vi "MOCVD_Growth_Sequence_Editor.vi"() -> ()   [LabVIEW 2011]
doc: "This is the top-level Growth Sequence Editor Application, and the only VI that needs to be executed by the end-user to edit and run a growth sequence. This application provides all functions necessary for opening, saving, and editing growth sequence files."
uses:
  low_level_proc/globals.vi
panel:
  out "opening_sequence":bool
  out "Error Out":errorcluster
  out "Total Time":string caption="Total Growth Time:"
  out "Notes":string
  out "Growth Name":string
  out "Operator Name":string
  out "Db Info Set":bool
  in  "Set DB Info":bool
  out "Use Database":bool=TRUE
  out "Log Files Directory":path=path "C:/MOCVD/Log Files"
  in  "Preferences":bool
  in  "Iterations":u32=1 min=1
  out "Delete Event":bool
  out "Current File Path":path
  in  "Save":bool
  out "Application Name":string
  in  "Comment":string
  out "Error Out":errorcluster caption="error out"
  in  "Operating Mode":enum32{"Production", "Debug"}(radio)=enum."Debug"
  in  "View Log":bool
  in  "Resume":bool
  in  "Exit":bool
  in  "New Sequence":bool
  in  "Save As":bool
  in  "Command Tabs":T1(tab)
  in  "Active":bool
  in  "Run":bool
  in  "Flow 1":dbl caption="Flow 1 (sccm)" min=0.0
  in  "Flow 2":dbl caption="Flow 2 (sccm)" min=0.0
  in  "Flow 3":dbl caption="Flow 3 (sccm)" min=0.0
  in  "Flow 4":dbl caption="Flow 4 (sccm)" min=0.0
  in  "Gas_Source_In":bool caption="Gas Source In"
  in  "H2 Flush":bool
  in  "Bubbler In":bool
  in  "H2_Dilute":bool caption="H2 Dilute"
  in  "Remote Flow":bool caption="Remote"
  in  "Spinner":bool
  in  "Heater":bool
  in  "Remote Heater":bool caption="Remote"
  in  "Atm_Exhaust":bool
  in  "Vac_Exhaust":bool
  in  "Remote Vacuum":bool caption="Remote"
  in  "Prompt":string
  in  "API Front Panel":bool
  in  "Move Down":bool
  in  "Move Up":bool
  in  "Copy Event":bool
  in  "Time (s)":dbl min=0.0
  out "Command":string
  in  "Command Sequence":i32[](listbox)
  in  "Delete Event":bool
  in  "Insert Event":bool
  in  "Run Sequence":bool
  in  "Open Sequence":bool
  # "Wait for user input before continuing sequence"
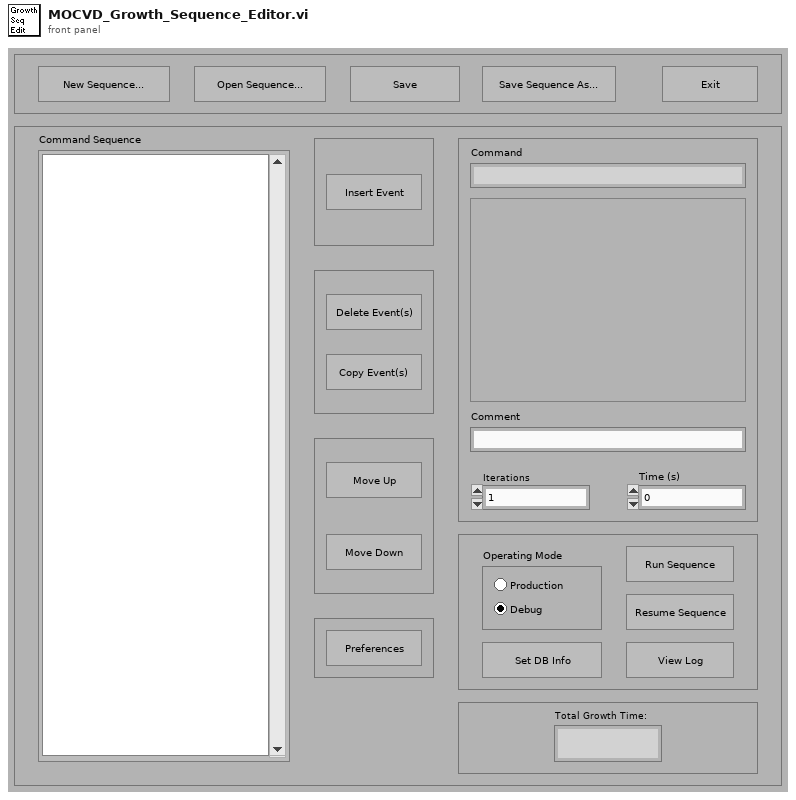
[diagram p1: front panel]
types:
  T1 = enum32{"Default", "Flow", "Heater", "Vacuum", "Wait", "API"}
  T2 = cluster{"Command":string, "Argument List":string[], dbl[], "element":dbl}
  T3 = cluster{"Command":string, "Argument List Out":string[], dbl[], "element":dbl}
  T4 = cluster{"Command":string, string[], dbl[], "element":dbl}
  T5 = enum16{"Discrete", "Continuous", "Instantaneous", "Finite"}
  T6 = cluster{string, "Argument List Out":string[], dbl[], dbl}
  T7 = enum8{"Enabled", "Disabled", "Disabled and Grayed Out"}
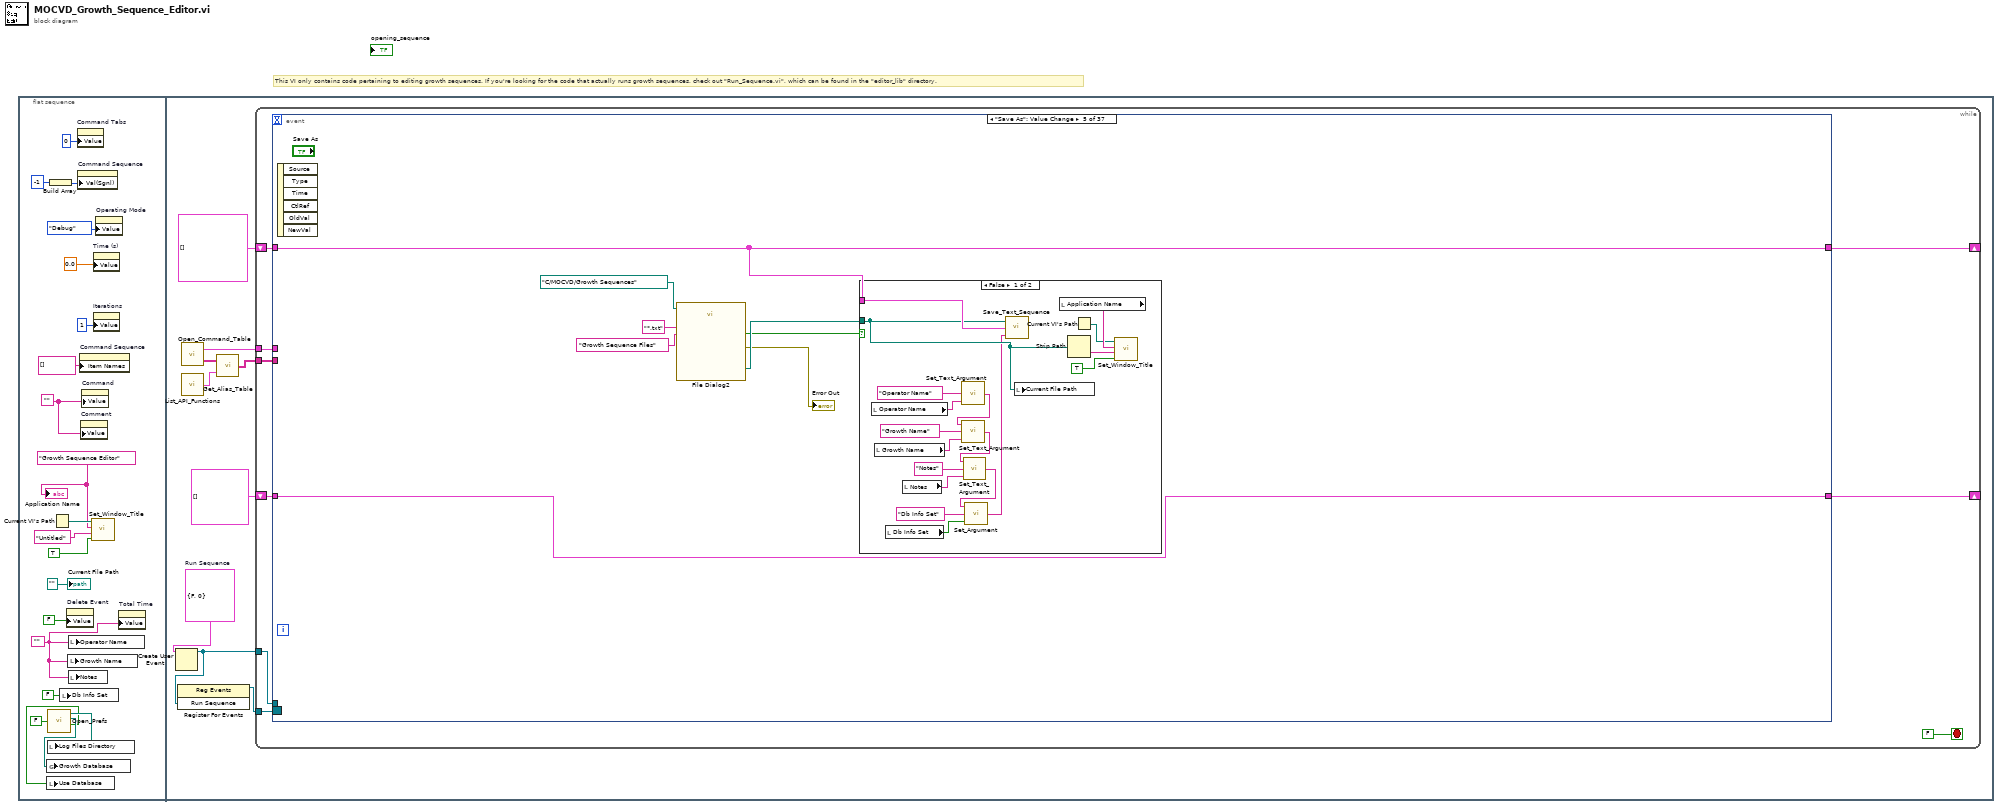
[diagram p0: block diagram]
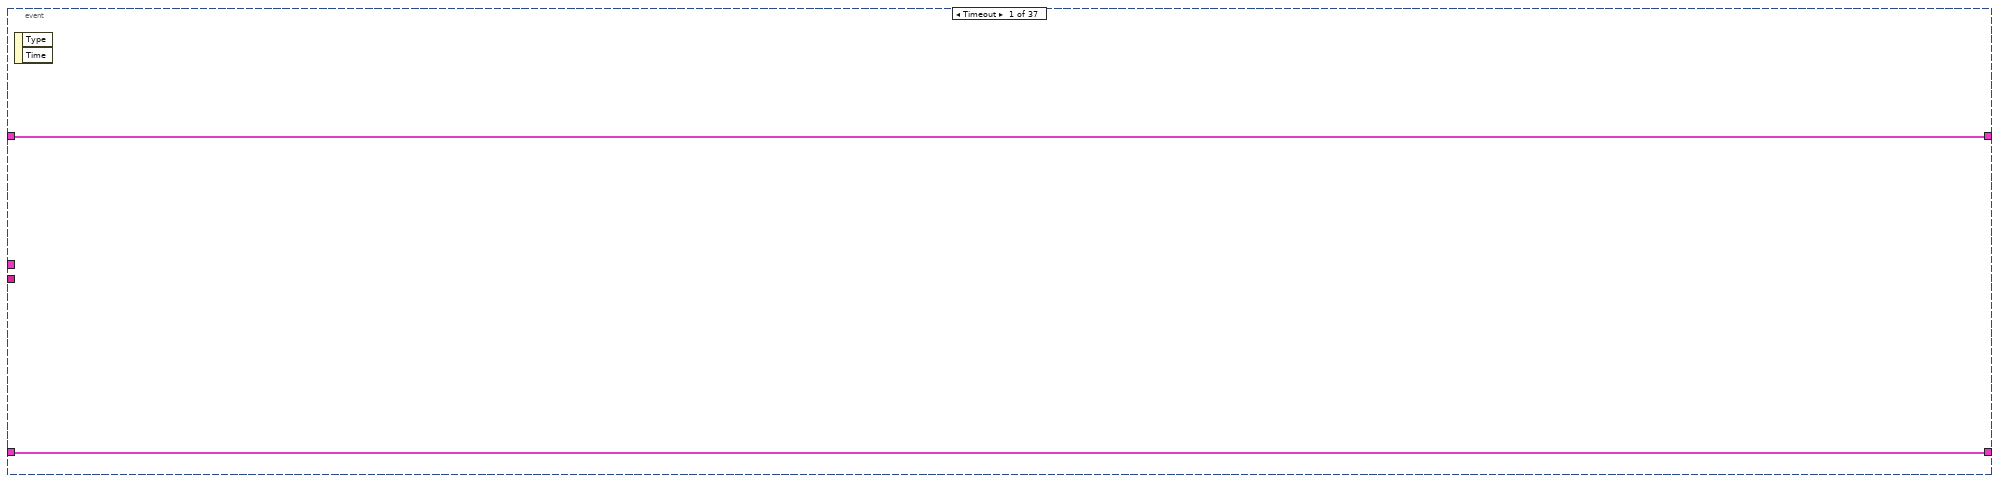
[diagram p2: hidden frame]
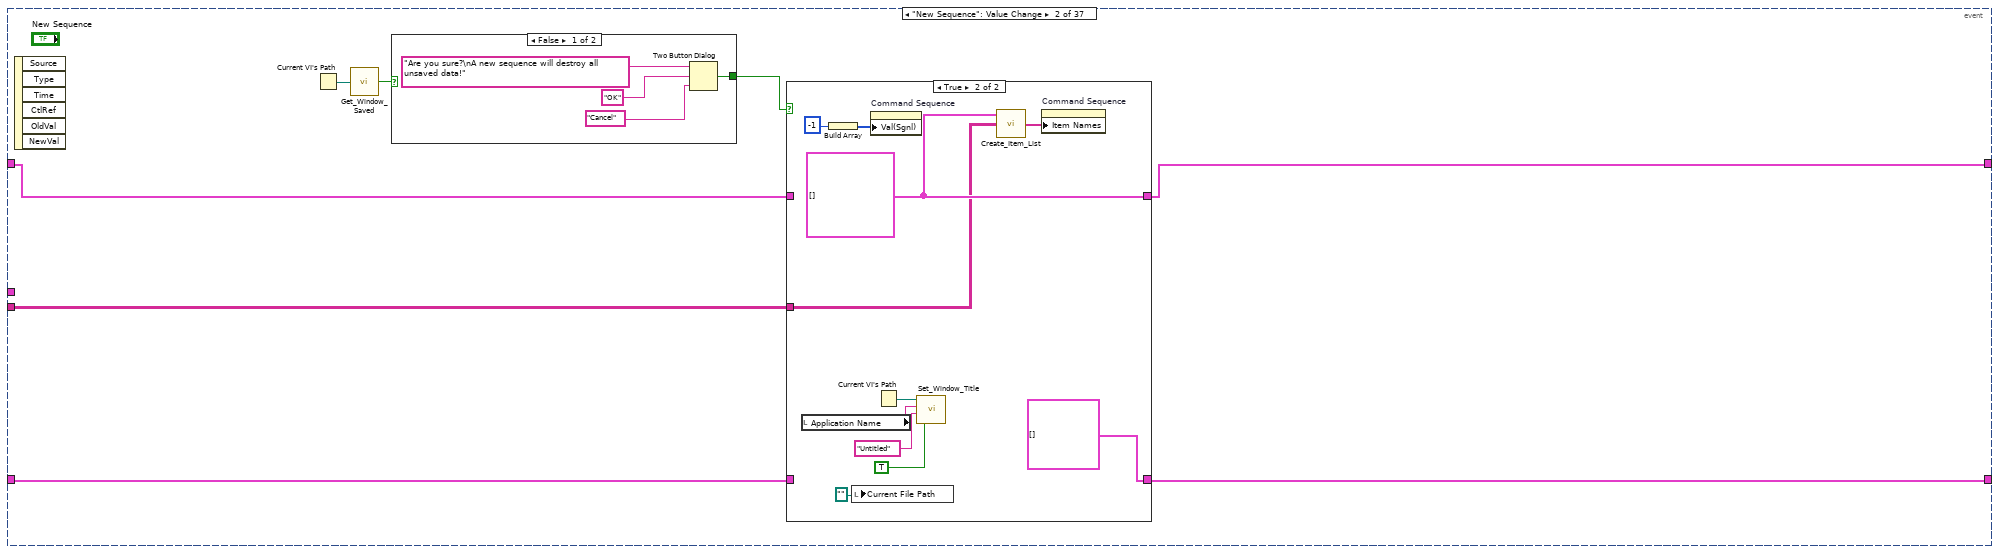
[diagram p3: hidden frame]
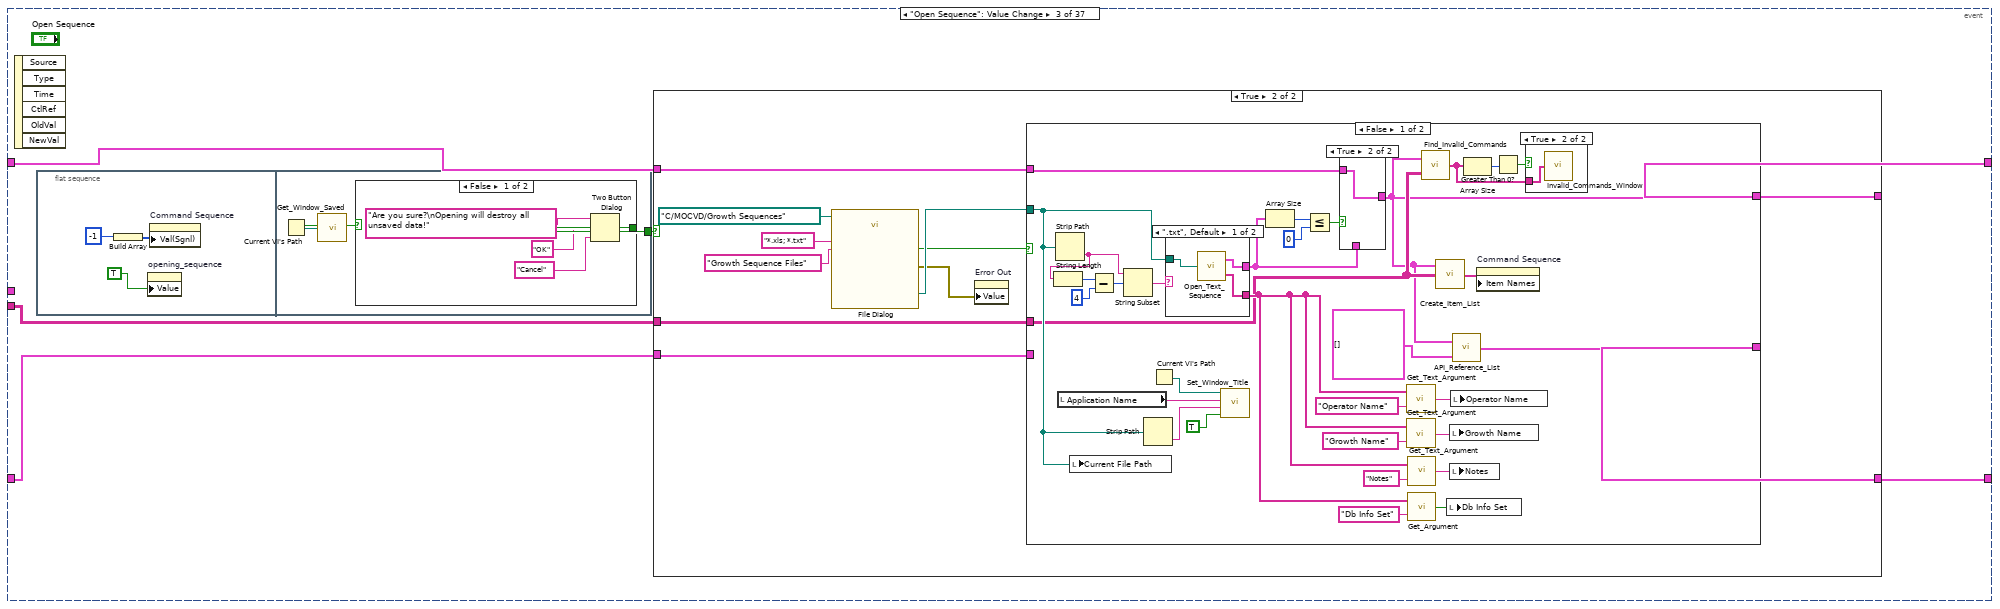
[diagram p6: hidden frame]
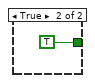
[diagram p7: hidden frame]
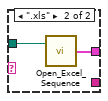
[diagram p10: hidden frame]
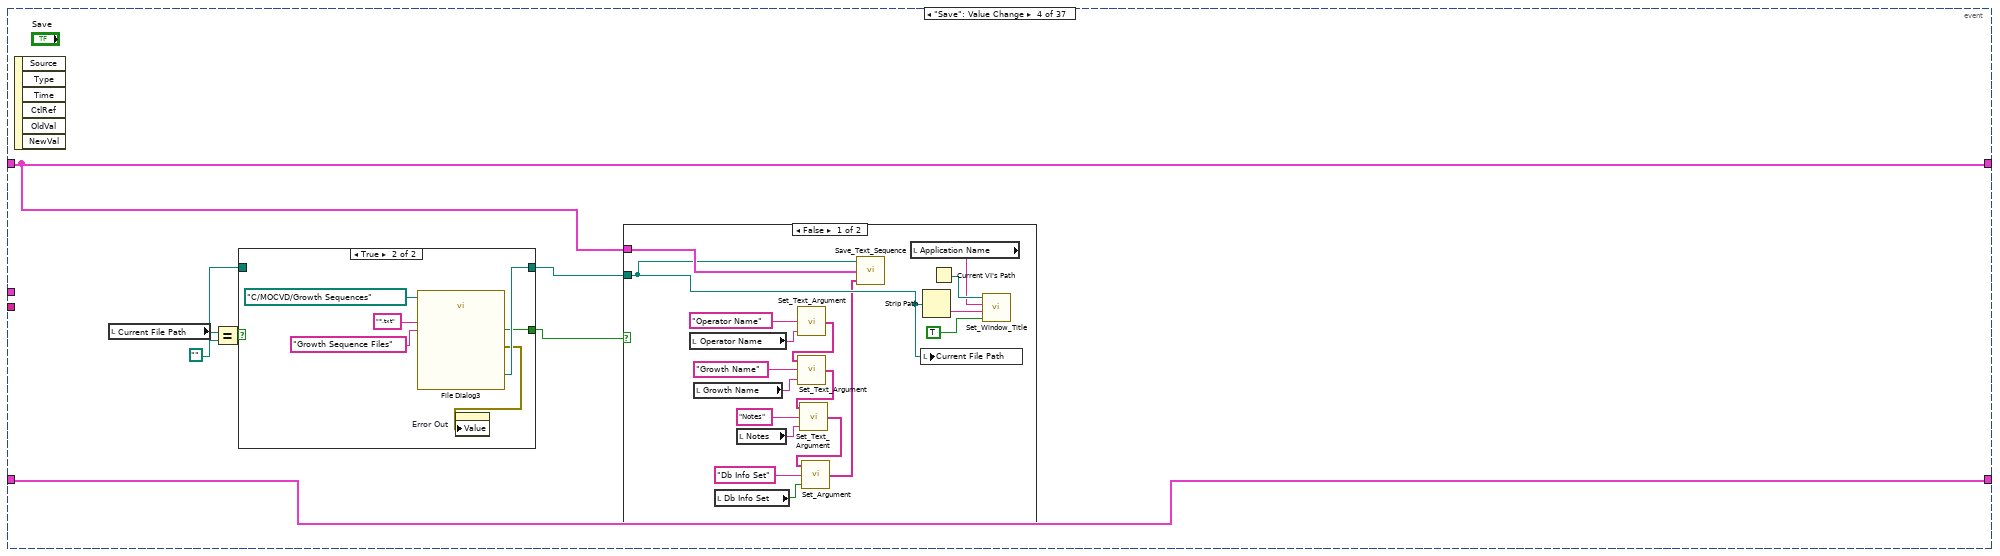
[diagram p13: hidden frame]
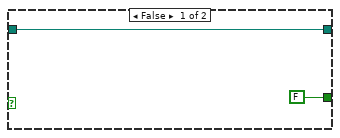
[diagram p14: hidden frame]
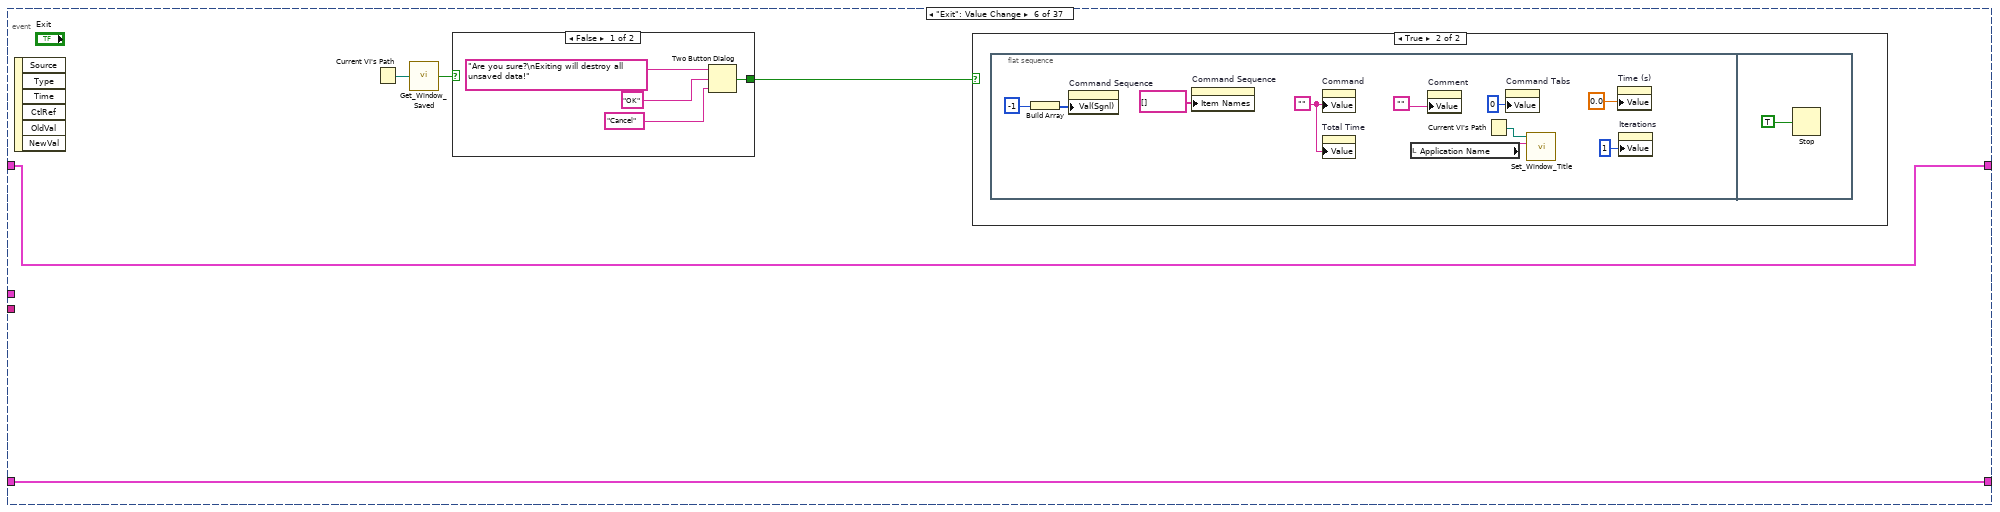
[diagram p17: hidden frame]
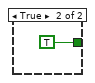
[diagram p18: hidden frame]
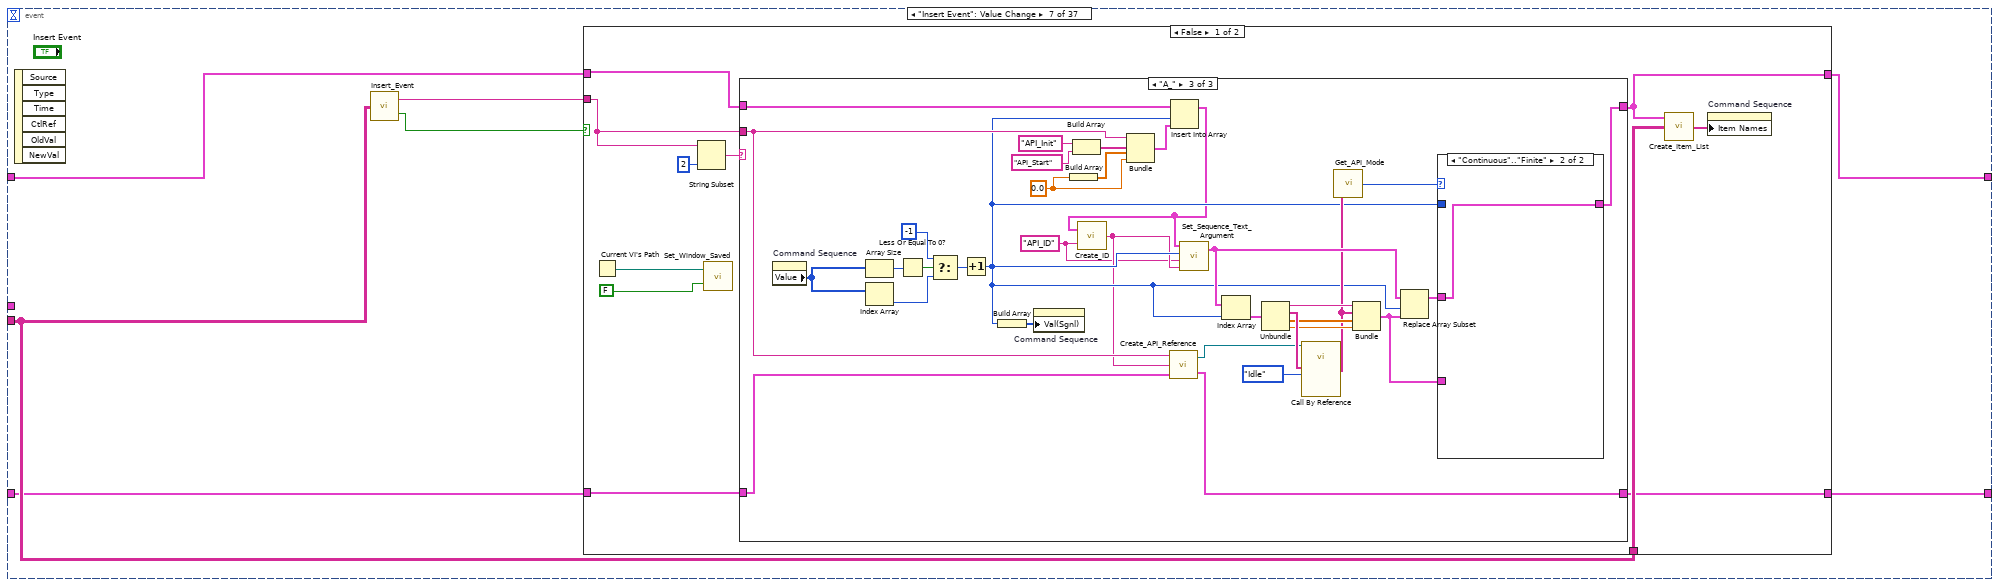
[diagram p20: hidden frame]
diagram:
  # "This VI only contains code pertaining to editing growth sequences. If you're looking for the code that actually runs growth sequences, check out \"Run_Sequence.vi\", which can be found in the \"editor_lib\" directory."
  n1 = flat-sequence {
    frame #0 {
      w1 = ""
      w15 = "Growth Sequence Editor" ("Application Title")
      w17 = ""
      n2 = call "Open_Prefs.vi"("Open Window"=FALSE) -> ("Log Files Directory Out"=w5:path, "MOCVD Database File Out"=w4:path, "Use Database Out"=w3:bool)  [unwired: 1 out]
      n3 = global write "globals.vi" "Growth Database"(w4) -> ()
      n4 = local write "Use Database"(w3) -> ()
      n5 = local write "Log Files Directory"(w5) -> ()
      n6 = Build Array(-1) -> (w8:i32[])
      n7 = Current VI's Path() -> (path=w16:path)
      n8 = local write "Db Info Set"(FALSE ("Db Info Set")) -> ()
      n9 = property on="Delete Event" class="Bool (strict)"("Value"=FALSE ("Delete Event")) -> ()  [unwired: 2 in, 2 out]
      n10 = local write "Growth Name"(w1) -> ()
      n11 = local write "Operator Name"(w1) -> ()
      n12 = local write "Notes"(w1) -> ()
      n13 = property on="Command Tabs" class="TabCtl (strict)"("Value"=0) -> ()  [unwired: 2 in, 2 out]
      n14 = property on="Command Sequence" class="LstBox (strict)"("Val(Sgnl)"=w8) -> ()  [unwired: 2 in, 2 out]
      n15 = property on="Command Sequence" class="LstBox (strict)"("Item Names"=string[] []) -> ()  [unwired: 2 in, 2 out]
      n16 = property on="Comment" class="Str"("Value"=w17) -> ()  [unwired: 2 in, 2 out]
      n17 = property on="Command" class="Str"("Value"=w17) -> ()  [unwired: 2 in, 2 out]
      n18 = call "Set_Window_Title.vi"("Saved"=TRUE, "Current File"="Untitled", "Application Name"=w15, "VI Path"=w16) -> ()  [unwired: 1 out]
      n19 = property on="Time (s)" class="DigNum (strict)"("Value"=0.0 ("Flow1")) -> ()  [unwired: 2 in, 2 out]
      n20 = property on="Iterations" class="DigNum (strict)"("Value"=u32 1 ("Repetitions")) -> ()  [unwired: 2 in, 2 out]
      n21 = property on="Operating Mode" class="RadioBtnsControl (strict)"("Value"=enum32{"Production", "Debug"}."Debug" ("Operating Mode")) -> ()  [unwired: 2 in, 2 out]
      n22 = property on="Total Time" class="Str"("Value"=w1) -> ()  [unwired: 2 in, 2 out]
      "Application Name" <- w15
      "Current File Path" <- path ""
    }
    frame #1 {
      w28 = cluster{"Resume":bool, "Start Event":i32} {"Resume"=FALSE, "Start Event"=0}  # Run Sequence
      n23 = Create User Event(user event datatype=w28) -> (user event=w26:refnum<user-event>)  [unwired: 1 in, 1 out]
      n24 = register-events(w26) -> (reference out=w27:refnum<event-registration>)  [unwired: 2 in, 1 out]
      n25 = call "Open_Command_Table.vi"() -> ("Commands"=w29:cluster{string, string[]}[], "Alias Table"=w25:string[][])  [unwired: 1 out]
      n26 = call "List_API_Functions.vi"() -> ("API Functions Table"=w23:cluster{string, string, path}[])  [unwired: 1 out]
      n27 = call "Get_Alias_Table.vi"("API Functions Table"=w23, "Alias Table In"=w25) -> ("Alias Table Out"=w24:string[][])
      n28 = while {
        shift-right: [w36] -> _
        shift-left: cluster{string, string[], dbl[], dbl}[] [] ("Output Sequence") -> [w37]
        tunnel: w29 -> [w35]
        tunnel: w27 -> [w34]
        tunnel: w26 -> [w33]
        tunnel: w24 -> [w32]
        shift-right: [w30] -> _
        shift-left: cluster{string, "VI Reference":refnum<vi>}[] [] ("API Function Array") -> [w31]
        stop <- FALSE stop-if-true
        n29 = event shown="[4] \"Save As\": Value Change" {
          selector: w34 -> [_ _ _ _ _ _ _ _ _ _ _ _ _ _ _ _ _ _ _ _ _ _ _ _ _ _ _ _ _ _ _ _ _ _ _ _ _]
          dyn-events: _ -> [_ _ _ _ _ _ _ _ _ _ _ _ _ _ _ _ _ _ _ _ _ _ _ _ _ _ _ _ _ _ _ _ _ _ _ _ _]
          timeout: _ -> [_ _ _ _ _ _ _ _ _ _ _ _ _ _ _ _ _ _ _ _ _ _ _ _ _ _ _ _ _ _ _ _ _ _ _ _ _]
          tunnel: w37 -> [w40 w47 w72 w144 w175 w202 w225 w345 w435 w472 w503 w523 w536 w545 w772 w776 w783 w787 w797 w806 w815 w824 w833 w842 w851 w860 w870 w879 w888 w897 w906 w911 w935 w952 w955 w995 w1018]
          tunnel: [w40 w46 w71 w144 w175 w202 w224 w350 w434 w463 w489 w523 w536 w542 w772 w776 w783 w787 w795 w804 w813 w822 w831 w840 w849 w858 w868 w877 w886 w895 w904 w911 w927 w952 w954 w995 w1018] -> w36
          tunnel: w35 -> [_ _ _ _ _ _ _ _ _ _ _ _ _ w555 _ _ _ _ _ _ _ _ _ _ _ _ _ _ _ _ _ _ _ _ _ _ _]
          tunnel: w33 -> [_ _ _ _ _ _ _ _ _ _ _ _ _ _ _ _ _ _ _ _ _ _ _ _ _ _ _ _ _ _ _ _ _ _ w964 w999 _]
          tunnel: w32 -> [_ w45 w70 _ _ _ w221 w342 w430 w469 w496 _ _ w551 _ _ _ _ _ _ _ _ _ _ _ _ _ _ _ _ _ _ w930 _ _ w997 w1013]
          tunnel: w31 -> [w39 w44 w69 w145 w172 w200 w219 w341 w429 w468 w495 w524 w535 w550 w771 w774 w782 w786 w791 w800 w809 w818 w827 w836 w845 w854 w864 w873 w882 w891 w900 w909 w931 w951 w963 w996 w1011]
          tunnel: [w39 w43 w68 w145 w172 w200 w220 w340 w428 w468 w495 w524 w535 w549 w771 w774 w782 w786 w791 w800 w809 w818 w827 w836 w845 w854 w864 w873 w882 w891 w900 w909 w931 w951 w963 w996 w1011] -> w30
          event Timeout {
            n30 = event-data() -> ()  [unwired: 3 out]
          }
          event "New Sequence": Value Change {
            n31 = event-data() -> ()  [unwired: 7 out]
            n32 = Current VI's Path() -> (path=w42:path)
            n33 = call "Get_Window_Saved.vi"("VI Path"=w42) -> ("Saved"=w41:bool)
            n34 = case shown="False" w41 {
              selector: w41 -> [_ w53]
              tunnel: [w49 w53] -> w48
              frame False {
                n35 = Two Button Dialog(message="Are you sure?\nA new sequence will destroy all unsaved data!", 1:"Cancel" ("F button name (\"Cancel\")"), 2:"OK" ("T button name (\"OK\")")) -> (T button?=w49:bool)
              }
              frame True {
              }
            }
            n36 = case shown="True" w48 {
              tunnel: w47 -> [w55 _]
              tunnel: [w55 w66] -> w46
              tunnel: w45 -> [_ w62]
              tunnel: w44 -> [w54 _]
              tunnel: [w54 cluster{string, "VI Reference":refnum<vi>}[] [] ("API Function Array")] -> w43
              frame False {
              }
              frame True {
                w66 = cluster{string, string[], dbl[], dbl}[] [] ("Output Sequence")
                n37 = local read "Application Name"() -> (w59:string)
                n38 = Build Array(-1 ("Value (Signaling)")) -> (w63:i32[])
                n39 = local write "Current File Path"(path "") -> ()
                n40 = property on="Command Sequence" class="LstBox (strict)"("Val(Sgnl)"=w63) -> ()  [unwired: 2 in, 2 out]
                n41 = Current VI's Path() -> (path=w60:path)
                n42 = call "Set_Window_Title.vi"("Saved"=TRUE, "Current File"="Untitled", "Application Name"=w59, "VI Path"=w60) -> ()  [unwired: 1 out]
                n43 = call "Create_Item_List.vi"("Alias Table"=w62, "Sequence"=w66) -> ("Item List"=w65:string[])  [unwired: 1 in]
                n44 = property on="Command Sequence" class="LstBox (strict)"("Item Names"=w65) -> ()  [unwired: 2 in, 2 out]
              }
            }
          }
          event "Open Sequence": Value Change {
            n45 = event-data() -> ()  [unwired: 7 out]
            n46 = flat-sequence {
              tunnel: [w76] -> w67
              frame #0 {
                n47 = Build Array(-1 ("Value (Signaling)")) -> (w74:i32[])
                n48 = property on="opening_sequence" class="Bool (strict)"("Value"=TRUE ("opening_sequence")) -> ()  [unwired: 2 in, 2 out]
                n49 = property on="Command Sequence" class="LstBox (strict)"("Val(Sgnl)"=w74) -> ()  [unwired: 2 in, 2 out]
              }
              frame #1 {
                n50 = Current VI's Path() -> (path=w78:path)
                n51 = call "Get_Window_Saved.vi"("VI Path"=w78) -> ("Saved"=w77:bool)
                n52 = case shown="False" w77 {
                  tunnel: [w79 TRUE ("T button?")] -> w76
                  frame False {
                    n53 = Two Button Dialog(message="Are you sure?\nOpening will destroy all unsaved data!", 1:"Cancel" ("F button name (\"Cancel\")"), 2:"OK" ("T button name (\"OK\")")) -> (T button?=w79:bool)
                  }
                  frame True {
                  }
                }
              }
            }
            n54 = case shown="True" w67 {
              tunnel: w72 -> [w85 w96]
              tunnel: [w85 w95] -> w71
              tunnel: w70 -> [_ w88]
              tunnel: w69 -> [w84 w87]
              tunnel: [w84 w86] -> w68
              frame False {
              }
              frame True {
                n55 = call "File Dialog"("start path"=path "C:/MOCVD/Growth Sequences", "pattern (all files)"="*.xls; *.txt" ("pattern label"), "pattern label"="Growth Sequence Files") -> ("selected path"=w94:path, "cancelled"=w93:bool, "error out"=w89:errorcluster)  [unwired: 4 in, 6 out]
                n56 = property on="Error Out" class="Clust (strict)"("Value"=w89) -> ()  [unwired: 2 in, 2 out]
                n57 = case shown="False" w93 {
                  tunnel: w96 -> [w125 w138]
                  tunnel: [w100 w138] -> w95
                  tunnel: w94 -> [w113 _]
                  tunnel: w88 -> [w101 _]
                  tunnel: w87 -> [_ w137]
                  tunnel: [w117 w137] -> w86
                  frame False {
                    n58 = Strip Path(path=w113) -> (name=w122:string)  [unwired: 1 out]
                    n59 = String Length(string=w122) -> (length=w121:i32)
                    n60 = local read "Application Name"() -> (w116:string)
                    n61 = local write "Current File Path"(w113) -> ()
                    n62 = Subtract(x=w121, y=4) -> (x-y=w119:i32)
                    n63 = String Subset(string=w122, offset (0)=w119) -> (substring=w118:string)  [unwired: 1 out]
                    n64 = Strip Path(path=w113) -> (name=w115:string)  [unwired: 1 out]
                    n65 = Current VI's Path() -> (path=w102:path)
                    n66 = case shown="\".txt\", Default" w118 {
                      tunnel: [w132 w134] -> w124
                      tunnel: w113 -> [w131 w133]
                      tunnel: [w130 _] -> w106
                      frame ".txt", Default {
                        n67 = call "Open_Text_Sequence.vi"("Text File"=w131) -> ("Sequence"=w132:cluster{string, string[], dbl[], dbl}[], "Header"=w130:string[])
                      }
                      frame ".xls" {
                        n68 = call "Open_Excel_Sequence.vi"("Excel File Path"=w133) -> ("Sequence"=w134:cluster{string, string[], dbl[], dbl}[])  [unwired: 1 in]
                      }
                    }
                    n69 = call "Set_Window_Title.vi"("Saved"=TRUE, "Current File"=w115, "Application Name"=w116, "VI Path"=w102) -> ()  [unwired: 1 out]
                    n70 = Array Size(array=w124) -> (size(s)=w128:i32)
                    n71 = Less Or Equal?(x=w128, y=0) -> (x <= y?=w126:bool)
                    n72 = case shown="True" w126 {
                      tunnel: w125 -> [_ w136]
                      tunnel: w124 -> [w135 _]
                      tunnel: [w135 w136] -> w100
                      frame False {
                      }
                      frame True {
                      }
                    }
                    n73 = call "Get_Text_Argument.vi"("Argument"="Operator Name", "Argument List"=w106) -> ("Text"=w111:string)
                    n74 = call "Get_Text_Argument.vi"("Argument"="Growth Name", "Argument List"=w106) -> ("Text"=w109:string)
                    n75 = call "Get_Text_Argument.vi"("Argument"="Notes", "Argument List"=w106) -> ("Text"=w108:string)
                    n76 = call "Get_Argument.vi"("Argument"="Db Info Set", "Argument List"=w106) -> ("Enabled"=w104:bool)
                    n77 = call "Find_Invalid_Commands.vi"("Alias Table"=w101, "Input Sequence"=w100) -> ("Invalid Commands"=w97:string[])
                    n78 = call "Create_Item_List.vi"("Alias Table"=w101, "Sequence"=w100) -> ("Item List"=w123:string[])  [unwired: 1 in]
                    n79 = local write "Db Info Set"(w104) -> ()
                    n80 = local write "Growth Name"(w109) -> ()
                    n81 = local write "Notes"(w108) -> ()
                    n82 = local write "Operator Name"(w111) -> ()
                    n83 = call "API_Reference_List.vi"("API Function Array In"=cluster{string, "VI Reference":refnum<vi>}[] [] ("API Function Array"), "Command Sequence"=w100) -> ("API Function Array Out"=w117:cluster{string, "VI Reference":refnum<vi>}[])
                    n84 = Array Size(array=w97) -> (size(s)=w99:i32)
                    n85 = property on="Command Sequence" class="LstBox (strict)"("Item Names"=w123) -> ()  [unwired: 2 in, 2 out]
                    n86 = Greater Than 0?(x=w99) -> (x > 0?=w98:bool)
                    n87 = case shown="True" w98 {
                      tunnel: w97 -> [_ w129]
                      frame False {
                      }
                      frame True {
                        n88 = call "Invalid_Commands_Window.vi"("Invalid Commands"=w129) -> ()  [unwired: 1 in]
                      }
                    }
                  }
                  frame True {
                  }
                }
              }
            }
          }
          event "Save": Value Change {
            n89 = event-data() -> ()  [unwired: 7 out]
            n90 = local read "Current File Path"() -> (w139:path)
            n91 = Equal?(x=w139, y=path "") -> (x = y?=w141:bool)
            n92 = case shown="True" w141 {
              tunnel: [w146 w150] -> w142
              tunnel: [FALSE ("cancelled") w148] -> w140
              tunnel: w139 -> [w146 _]
              frame False {
              }
              frame True {
                n93 = call "File Dialog3"("start path"=path "C:/MOCVD/Growth Sequences", "pattern (all files)"="*.txt" ("pattern label"), "pattern label"="Growth Sequence Files") -> ("selected path"=w150:path, "cancelled"=w148:bool, "error out"=w149:errorcluster)  [unwired: 4 in, 6 out]
                n94 = property on="Error Out" class="Clust (strict)"("Value"=w149) -> ()  [unwired: 2 in, 2 out]
              }
            }
            n95 = case shown="False" w140 {
              tunnel: w142 -> [w158 _]
              tunnel: w144 -> [w171 _]
              frame False {
                n96 = local read "Operator Name"() -> (w159:string)
                n97 = local read "Growth Name"() -> (w163:string)
                n98 = local read "Db Info Set"() -> (w154:bool)
                n99 = local read "Notes"() -> (w166:string)
                n100 = call "Set_Text_Argument.vi"("Text"=w159, "Argument"="Operator Name") -> ("Argument List Out"=w161:string[])  [unwired: 1 in]
                n101 = call "Set_Text_Argument.vi"("Text"=w163, "Argument"="Growth Name", "Argument List In"=w161) -> ("Argument List Out"=w164:string[])
                n102 = call "Set_Text_Argument.vi"("Text"=w166, "Argument"="Notes", "Argument List In"=w164) -> ("Argument List Out"=w157:string[])
                n103 = call "Set_Argument.vi"("Enable"=w154, "Argument"="Db Info Set", "Argument List In"=w157) -> ("Argument List Out"=w156:string[])
                n104 = call "Save_Text_Sequence.vi"("Header"=w156, "Sequence"=w171, "Text File"=w158) -> ()  [unwired: 1 in]
                n105 = local read "Application Name"() -> (w167:string)
                n106 = local write "Current File Path"(w158) -> ()
                n107 = Strip Path(path=w158) -> (name=w170:string)  [unwired: 1 out]
                n108 = Current VI's Path() -> (path=w169:path)
                n109 = call "Set_Window_Title.vi"("Saved"=TRUE, "Current File"=w170, "Application Name"=w167, "VI Path"=w169) -> ()  [unwired: 1 out]
              }
              frame True {
              }
            }
          }
          event "Save As": Value Change {
            n110 = event-data() -> ()  [unwired: 7 out]
            n111 = call "File Dialog2"("start path"=path "C:/MOCVD/Growth Sequences", "pattern (all files)"="*.txt" ("pattern label"), "pattern label"="Growth Sequence Files") -> ("selected path"=w176:path, "cancelled"=w174:bool, "error out"=→"Error Out":errorcluster)  [unwired: 4 in, 6 out]
            n112 = case shown="False" w174 {
              tunnel: w176 -> [w192 _]
              tunnel: w175 -> [w197 _]
              frame False {
                n113 = local read "Operator Name"() -> (w183:string)
                n114 = local read "Growth Name"() -> (w182:string)
                n115 = local read "Db Info Set"() -> (w180:bool)
                n116 = local read "Notes"() -> (w181:string)
                n117 = call "Set_Text_Argument.vi"("Text"=w183, "Argument"="Operator Name") -> ("Argument List Out"=w191:string[])  [unwired: 1 in]
                n118 = call "Set_Text_Argument.vi"("Text"=w182, "Argument"="Growth Name", "Argument List In"=w191) -> ("Argument List Out"=w186:string[])
                n119 = call "Set_Text_Argument.vi"("Text"=w181, "Argument"="Notes", "Argument List In"=w186) -> ("Argument List Out"=w189:string[])
                n120 = call "Set_Argument.vi"("Enable"=w180, "Argument"="Db Info Set", "Argument List In"=w189) -> ("Argument List Out"=w184:string[])
                n121 = call "Save_Text_Sequence.vi"("Header"=w184, "Sequence"=w197, "Text File"=w192) -> ()  [unwired: 1 in]
                n122 = local write "Current File Path"(w192) -> ()
                n123 = local read "Application Name"() -> (w196:string)
                n124 = Strip Path(path=w192) -> (name=w195:string)  [unwired: 1 out]
                n125 = Current VI's Path() -> (path=w194:path)
                n126 = call "Set_Window_Title.vi"("Saved"=TRUE, "Current File"=w195, "Application Name"=w196, "VI Path"=w194) -> ()  [unwired: 1 out]
              }
              frame True {
              }
            }
          }
          event "Exit": Value Change {
            n127 = event-data() -> ()  [unwired: 7 out]
            n128 = Current VI's Path() -> (path=w199:path)
            n129 = call "Get_Window_Saved.vi"("VI Path"=w199) -> ("Saved"=w198:bool)
            n130 = case shown="False" w198 {
              tunnel: [w203 TRUE ("T button?")] -> w201
              frame False {
                n131 = Two Button Dialog(message="Are you sure?\nExiting will destroy all unsaved data!", 1:"Cancel" ("F button name (\"Cancel\")"), 2:"OK" ("T button name (\"OK\")")) -> (T button?=w203:bool)
              }
              frame True {
              }
            }
            n132 = case shown="True" w201 {
              frame False {
              }
              frame True {
                n133 = flat-sequence {
                  frame #0 {
                    w208 = ""
                    n134 = Build Array(-1 ("Command Sequence")) -> (w215:i32[])
                    n135 = property on="Command Sequence" class="LstBox (strict)"("Val(Sgnl)"=w215) -> ()  [unwired: 2 in, 2 out]
                    n136 = property on="Command Sequence" class="LstBox (strict)"("Item Names"=string[] []) -> ()  [unwired: 2 in, 2 out]
                    n137 = property on="Command" class="Str"("Value"=w208) -> ()  [unwired: 2 in, 2 out]
                    n138 = property on="Total Time" class="Str"("Value"=w208) -> ()  [unwired: 2 in, 2 out]
                    n139 = local read "Application Name"() -> (w212:string)
                    n140 = property on="Comment" class="Str"("Value"="") -> ()  [unwired: 2 in, 2 out]
                    n141 = Current VI's Path() -> (path=w211:path)
                    n142 = property on="Command Tabs" class="TabCtl (strict)"("Value"=0) -> ()  [unwired: 2 in, 2 out]
                    n143 = call "Set_Window_Title.vi"("Application Name"=w212, "VI Path"=w211) -> ()  [unwired: 2 in, 1 out]
                    n144 = property on="Time (s)" class="DigNum (strict)"("Value"=0.0 ("Time (s)")) -> ()  [unwired: 2 in, 2 out]
                    n145 = property on="Iterations" class="DigNum (strict)"("Value"=u32 1 ("Repetitions")) -> ()  [unwired: 2 in, 2 out]
                  }
                  frame #1 {
                    n146 = Stop(stop? (T)=TRUE) -> ()
                  }
                }
              }
            }
          }
          event "Insert Event": Value Change {
            n147 = event-data() -> ()  [unwired: 7 out]
            n148 = call "Insert_Event.vi"("Alias Table"=w221) -> ("Command"=w223:string, "Cancelled"=w222:bool)
            n149 = case shown="False" w222 {
              tunnel: w225 -> [w236 w336]
              tunnel: [w234 w336] -> w224
              tunnel: w223 -> [w232 _]
              tunnel: w221 -> [w233 _]
              tunnel: [w230 w335] -> w220
              tunnel: w219 -> [w229 w335]
              frame False {
                n150 = Current VI's Path() -> (path=w228:path)
                n151 = String Subset(string=w232, length (rest)=2 ("length (rest)")) -> (substring=w226:string)  [unwired: 1 out]
                n152 = call "Set_Window_Saved.vi"("Saved"=FALSE, "VI Path"=w228) -> ()  [unwired: 1 out]
                n153 = case shown="\"A_\"" w226 {
                  tunnel: w236 -> [w253 w256 w313]
                  tunnel: [w239 w262 w291] -> w234
                  tunnel: w232 -> [w238 w267 w301]
                  tunnel: [w242 w277 w299] -> w230
                  tunnel: w229 -> [w242 w277 w300]
                  frame Default {
                    w251 = 0.0 ("element")
                    n154 = property on="Command Sequence" class="LstBox (strict)"() -> ("Value"=w247:i32[])  [unwired: 2 in, 2 out]
                    n155 = Array Size(array=w247) -> (size(s)=w243:i32)
                    n156 = Index Array(array=w247) -> (element=w245:i32)  [unwired: 1 in]
                    n157 = Less Or Equal To 0?(x=w243) -> (x <= 0?=w248:bool)
                    n158 = Select(t=-1, s=w248, f=w245) -> (s? t:f=w244:i32)
                    n159 = Increment(x=w244) -> (x+1=w249:i32)
                    n160 = Build Array(w249) -> (w250:i32[])
                    n161 = property on="Command Sequence" class="LstBox (strict)"("Val(Sgnl)"=w250) -> ()  [unwired: 2 in, 2 out]
                    n162 = call "Generate_Argument_List.vi"("Command"=w238) -> ("Argument List"=w237:string[])
                    n163 = Initialize Array(w251) -> (w252:dbl[])  [unwired: 1 out]
                    n164 = Increment(x=w244) -> (x+1=w240:i32)
                    n165 = Bundle("Command"=w238, "Argument List"=w237, w252, "element"=w251) -> (w241:T2)  [unwired: 1 out]
                    n166 = Insert Into Array(array=w253, index=w240, new element=w241) -> (w239:cluster{string, string[], dbl[], dbl}[])
                  }
                  frame "L_" {
                    w255 = "API_Loop_ID" ("Argument")
                    w254 = "API_ID" ("Argument")
                    w272 = 0.0 ("element")
                    n167 = property on="Command Sequence" class="LstBox (strict)"() -> ("Value"=w282:i32[])  [unwired: 2 in, 2 out]
                    n168 = Array Size(array=w282) -> (size(s)=w278:i32)
                    n169 = Index Array(array=w282) -> (element=w280:i32)  [unwired: 1 in]
                    n170 = Less Or Equal To 0?(x=w278) -> (x <= 0?=w283:bool)
                    n171 = Select(t=-1, s=w283, f=w280) -> (s? t:f=w279:i32)
                    n172 = Increment(x=w279) -> (x+1=w284:i32)
                    n173 = Build Array(w284) -> (w285:i32[])
                    n174 = property on="Command Sequence" class="LstBox (strict)"("Val(Sgnl)"=w285) -> ()  [unwired: 2 in, 2 out]
                    n175 = call "Create_ID.vi"("ID Argument Name"=w255, "Input Sequence"=w256) -> ("ID"=w261:string)
                    n176 = call "Generate_Argument_List.vi"("Command"=w267) -> ("Argument List"=w260:string[])
                    n177 = call "Create_ID.vi"("ID Argument Name"=w254, "Input Sequence"=w256) -> ("ID"=w257:string)
                    n178 = call "Set_Text_Argument.vi"("Text"=w257, "Argument"=w254, "Argument List In"=w260) -> ("Argument List Out"=w259:string[])
                    n179 = call "Set_Text_Argument.vi"("Text"=w261, "Argument"=w255, "Argument List In"=w259) -> ("Argument List Out"=w258:string[])
                    n180 = call "Set_Argument.vi"("Enable"=TRUE, "Argument"="API_Start", "Argument List In"=w258) -> ("Argument List Out"=w273:string[])
                    n181 = Initialize Array(w272) -> (w271:dbl[])  [unwired: 1 out]
                    n182 = call "Set_Argument.vi"("Enable"=TRUE, "Argument"="API_End", "Argument List In"=w258) -> ("Argument List Out"=w268:string[])
                    n183 = Increment(x=w279) -> (x+1=w266:i32)
                    n184 = Bundle("Command"=w267, "Argument List Out"=w273, w271, "element"=w272) -> (w276:T3)  [unwired: 1 out]
                    n185 = Bundle("Command"=w267, "Argument List Out"=w268, w271, "element"=w272) -> (w263:T3)  [unwired: 1 out]
                    n186 = Insert Into Array(array=w256, index=w266, new element=w276) -> (w265:cluster{string, string[], dbl[], dbl}[])
                    n187 = Increment(x=w266) -> (x+1=w264:i32)
                    n188 = Insert Into Array(array=w265, index=w264, new element=w263) -> (w262:cluster{string, string[], dbl[], dbl}[])
                  }
                  frame "A_" {
                    w286 = "API_ID" ("Argument")
                    w309 = 0.0 ("element")
                    n189 = property on="Command Sequence" class="LstBox (strict)"() -> ("Value"=w312:i32[])  [unwired: 2 in, 2 out]
                    n190 = Array Size(array=w312) -> (size(s)=w316:i32)
                    n191 = Index Array(array=w312) -> (element=w317:i32)  [unwired: 1 in]
                    n192 = Less Or Equal To 0?(x=w316) -> (x <= 0?=w318:bool)
                    n193 = Select(t=-1, s=w318, f=w317) -> (s? t:f=w314:i32)
                    n194 = Increment(x=w314) -> (x+1=w290:i32)
                    n195 = Build Array(w290) -> (w311:i32[])
                    n196 = property on="Command Sequence" class="LstBox (strict)"("Val(Sgnl)"=w311) -> ()  [unwired: 2 in, 2 out]
                    n197 = Build Array(w309) -> (w308:dbl[])
                    n198 = Build Array("API_Init" ("new element/subarray"), "API_Start" ("element")) -> (w310:string[])
                    n199 = Bundle("Command"=w301, w310, w308, "element"=w309) -> (w319:T4)  [unwired: 1 out]
                    n200 = Insert Into Array(array=w313, index=w290, new element=w319) -> (w288:cluster{string, string[], dbl[], dbl}[])
                    n201 = call "Create_ID.vi"("ID Argument Name"=w286, "Input Sequence"=w288) -> ("ID"=w287:string)
                    n202 = call "Create_API_Reference.vi"("API Function Array In"=w300, "ID"=w287, "Command"=w301) -> ("API Function Array Out"=w299:cluster{string, "VI Reference":refnum<vi>}[], "VI Reference"=w298:refnum<vi>)
                    n203 = call "Set_Sequence_Text_Argument.vi"("Text"=w287, "Argument"=w286, "Index"=w290, "Input Sequence"=w288) -> ("Output Sequence"=w296:cluster{string, string[], dbl[], dbl}[])  [unwired: 1 out]
                    n204 = Index Array(array=w296, index=w290) -> (element=w306:cluster{string, string[], dbl[], dbl})
                    n205 = Unbundle(w306) -> (w302:string, w305:string[], w304:dbl[], w303:dbl)
                    n206 = call-by-ref "?"(reference=w298, "State"=enum16{"Edit", "Start", "Run", "End", "Idle"}."Idle", "Argument List In"=w305) -> ("Argument List Out"=w294:string[])  [unwired: 3 in, 3 out]
                    n207 = call "Get_API_Mode.vi"("Argument List"=w294) -> ("API Mode"=w293:T5)
                    n208 = Bundle(w302, "Argument List Out"=w294, w304, w303) -> (w292:T6)  [unwired: 1 out]
                    n209 = Replace Array Subset(array=w296, new element=w292, index=w290) -> (w295:cluster{string, string[], dbl[], dbl}[])
                    n210 = case shown="\"Continuous\"..\"Finite\"" w293 {
                      tunnel: w295 -> [w325 w334]
                      tunnel: w290 -> [w333 _]
                      tunnel: w292 -> [w332 _]
                      tunnel: [w326 w334] -> w291
                      frame "Discrete", Default {
                        n211 = Increment(x=w333) -> (x+1=w320:i32)
                        n212 = Insert Into Array(array=w325, index=w320, new element=w332) -> (w324:cluster{string, string[], dbl[], dbl}[])
                        n213 = call "Set_Sequence_Argument.vi"("Enable"=FALSE, "Argument"="API_Start", "Index"=w320, "Input Sequence"=w324) -> ("Output Sequence"=w323:cluster{string, string[], dbl[], dbl}[])  [unwired: 1 out]
                        n214 = call "Set_Sequence_Argument.vi"("Enable"=TRUE, "Argument"="API_End", "Index"=w320, "Input Sequence"=w323) -> ("Output Sequence"=w327:cluster{string, string[], dbl[], dbl}[])  [unwired: 1 out]
                        n215 = call "Set_Sequence_Argument.vi"("Enable"=FALSE, "Argument"="API_Init", "Index"=w320, "Input Sequence"=w327) -> ("Output Sequence"=w326:cluster{string, string[], dbl[], dbl}[])  [unwired: 1 out]
                      }
                      frame "Continuous".."Finite" {
                      }
                    }
                  }
                }
                n216 = call "Create_Item_List.vi"("Alias Table"=w233, "Sequence"=w234) -> ("Item List"=w235:string[])  [unwired: 1 in]
                n217 = property on="Command Sequence" class="LstBox (strict)"("Item Names"=w235) -> ()  [unwired: 2 in, 2 out]
              }
              frame True {
              }
            }
          }
          event "Delete Event": Value Change {
            n218 = event-data() -> ()  [unwired: 7 out]
            n219 = Current VI's Path() -> (path=w339:path)
            n220 = call "Set_Window_Saved.vi"("Saved"=FALSE, "VI Path"=w339) -> ()  [unwired: 1 out]
            n221 = property on="Command Sequence" class="LstBox (strict)"() -> ("Value"=w348:i32[])  [unwired: 2 in, 2 out]
            n222 = Array Size(array=w348) -> (size(s)=w349:i32)
            n223 = Array Size(array=w345) -> (size(s)=w346:i32)
            n224 = Greater Than 0?(x=w349) -> (x > 0?=w343:bool)
            n225 = Greater Than 0?(x=w346) -> (x > 0?=w344:bool)
            n226 = And(x=w343, y=w344) -> (x .and. y?=w347:bool)
            n227 = case shown="True" w347 {
              tunnel: w345 -> [w352 w360]
              tunnel: [w352 w359] -> w350
              tunnel: w348 -> [_ w357]
              tunnel: w342 -> [_ w355]
              tunnel: w341 -> [w351 w354]
              tunnel: [w351 w353] -> w340
              frame False {
              }
              frame True {
                n228 = Index Array(array=w357) -> (element=w356:i32)  [unwired: 1 in]
                n229 = Greater Or Equal To 0?(x=w356) -> (x >= 0?=w358:bool)
                n230 = case shown="True" w358 {
                  tunnel: w360 -> [w362 w367]
                  tunnel: [w362 w366] -> w359
                  tunnel: w355 -> [_ w365]
                  tunnel: w354 -> [w361 w364]
                  tunnel: [w361 w363] -> w353
                  frame False {
                  }
                  frame True {
                    n231 = Two Button Dialog(message="Confirm event deletion?", 1:"Cancel" ("F button name (\"Cancel\")"), 2:"OK" ("T button name (\"OK\")")) -> (T button?=w371:bool)
                    n232 = case shown="True" w371 {
                      tunnel: w367 -> [w373 w374]
                      tunnel: [w373 w375] -> w366
                      tunnel: w365 -> [_ w387]
                      tunnel: w364 -> [w372 w384]
                      tunnel: [w372 w382] -> w363
                      frame False {
                      }
                      frame True {
                        n233 = property on="Command Sequence" class="LstBox (strict)"() -> ("Value"=w377:i32[])  [unwired: 2 in, 2 out]
                        n234 = call "Clean_Delete_Selection.vi"("Input Selection"=w377, "Input Sequence"=w374) -> ("Output Selection"=w376:i32[])
                        n235 = Sort 1D Array(array=w376) -> (sorted array=w392:i32[])
                        n236 = call "Delete_Commands.vi"("Command Indices"=w376, "Input Sequence"=w374) -> ("Output Sequence"=w375:cluster{string, string[], dbl[], dbl}[])
                        n237 = for {
                          tunnel: w392 -> [w413] mode=indexing
                          shift-right: [w415] -> w385
                          shift-left: string[] [] -> [w414]
                          tunnel: w374 -> [w412]
                          n238 = Index Array(array=w412, index=w413) -> (element=w421:cluster{string, string[], dbl[], dbl})
                          n239 = Unbundle(w421) -> (w420:string[])  [unwired: 3 out]
                          n240 = call "Get_Text_Argument.vi"("Argument"="API_ID", "Argument List"=w420) -> ("Text"=w416:string)
                          n241 = Not Equal?(x=w416, y="") -> (x != y?=w417:bool)
                          n242 = case shown="True" w417 {
                            tunnel: w416 -> [_ w425]
                            tunnel: [w422 w424] -> w415
                            tunnel: w414 -> [w422 w423]
                            frame False {
                            }
                            frame True {
                              n243 = Build Array (concatenate)(w425, w423) -> (w424:string[])
                            }
                          }
                        }
                        n244 = call "Create_Item_List.vi"("Alias Table"=w387, "Sequence"=w375) -> ("Item List"=w391:string[])  [unwired: 1 in]
                        n245 = property on="Command Sequence" class="LstBox (strict)"("Item Names"=w391) -> ()  [unwired: 2 in, 2 out]
                        n246 = for {
                          tunnel: w385 -> [w400]
                          tunnel: w384 -> [w394] mode=indexing
                          shift-right: [w393] -> w382
                          shift-left: cluster{string, "VI Reference":refnum<vi>}[] [] ("API Function Array") -> [w395]
                          n247 = Unbundle(w394) -> (w399:string, "VI Reference"=w396:refnum<vi>)
                          n248 = Search 1D Array(1D array=w400, element=w399) -> (index of element=w397:i32)  [unwired: 1 out]
                          n249 = Greater Or Equal To 0?(x=w397) -> (x >= 0?=w398:bool)
                          n250 = case shown="True" w398 {
                            tunnel: w396 -> [_ w406]
                            tunnel: w395 -> [w401 w405]
                            tunnel: w394 -> [w403 _]
                            tunnel: [w402 w405] -> w393
                            frame False {
                              n251 = Build Array (concatenate)(w401, w403) -> (w402:cluster{string, "VI Reference":refnum<vi>}[])
                            }
                            frame True {
                              n252 = Close Reference(reference=w406) -> (error out=→"Error Out":errorcluster)  [unwired: 1 in]
                            }
                          }
                        }
                        n253 = Array Size(array=w377) -> (size(s)=w390:i32)
                        n254 = Array Size(array=w375) -> (size(s)=w379:i32)
                        n255 = Greater Than 0?(x=w379) -> (x > 0?=w378:bool)
                        n256 = Equal?(x=1 ("y"), y=w390) -> (x = y?=w381:bool)
                        n257 = And(x=w378, y=w381) -> (x .and. y?=w380:bool)
                        n258 = case shown="True" w380 {
                          tunnel: w377 -> [_ w411]
                          tunnel: [i32[] [] ("Value (Signaling)") w408] -> w388
                          frame False {
                          }
                          frame True {
                            n259 = Index Array(array=w411) -> (element=w409:i32)  [unwired: 1 in]
                            n260 = Decrement(x=w409) -> (x-1=w410:i32)
                            n261 = Build Array(w410) -> (w408:i32[])
                          }
                        }
                        n262 = property on="Command Sequence" class="LstBox (strict)"("Val(Sgnl)"=w388) -> ()  [unwired: 2 in, 2 out]
                      }
                    }
                  }
                }
              }
            }
            "Delete Event" <- TRUE ("Delete Event")
          }
          event "Copy Event": Value Change {
            n263 = event-data() -> ()  [unwired: 7 out]
            n264 = Current VI's Path() -> (path=w427:path)
            n265 = call "Set_Window_Saved.vi"("Saved"=FALSE, "VI Path"=w427) -> ()  [unwired: 1 out]
            n266 = property on="Command Sequence" class="LstBox (strict)"() -> ("Value"=w431:i32[])  [unwired: 2 in, 2 out]
            n267 = Array Size(array=w431) -> (size(s)=w432:i32)
            n268 = Greater Than 0?(x=w432) -> (x > 0?=w433:bool)
            n269 = case shown="True" w433 {
              tunnel: w435 -> [w437 w440]
              tunnel: [w437 w453] -> w434
              tunnel: w431 -> [_ w441]
              tunnel: w430 -> [_ w445]
              tunnel: w429 -> [w436 w444]
              tunnel: [w436 w443] -> w428
              frame False {
              }
              frame True {
                n270 = call "Select_API_Commands.vi"("Input Selection"=w441, "Input Sequence"=w440) -> ("Output Selection"=w442:i32[])
                n271 = Array Size(array=w442) -> (size(s)=w451:i32)
                n272 = Decrement(x=w451) -> (x-1=w450:i32)
                n273 = Index Array(array=w442, index=w450) -> (element=w448:i32)
                n274 = Increment(x=w448) -> (x+1=w447:i32)
                n275 = for {
                  tunnel: w440 -> [w460]
                  tunnel: [w460] -> w439
                  tunnel: w442 -> [w459] mode=indexing
                  tunnel: [w458] -> w446 mode=indexing
                  tunnel: [w456] -> w452 mode=indexing
                  tunnel: w447 -> [w455]
                  tunnel: [w455] -> w449
                  i -> [w457]
                  n276 = Index Array(array=w460, index=w459) -> (element=w458:cluster{string, string[], dbl[], dbl})
                  n277 = Add(x=w455, y=w457) -> (x+y=w456:i32)
                }
                n278 = property on="Command Sequence" class="LstBox (strict)"("Val(Sgnl)"=w452) -> ()  [unwired: 2 in, 2 out]
                n279 = call "Copy_API_ID.vi"("Input List"=w446, "Input Sequence"=w439) -> ("Output List"=w438:cluster{string, string[], dbl[], dbl}[])
                n280 = Insert Into Array(array=w439, index=w449, new element=w438) -> (w453:cluster{string, string[], dbl[], dbl}[])
                n281 = call "API_Reference_List.vi"("API Function Array In"=w444, "Command Sequence"=w438) -> ("API Function Array Out"=w443:cluster{string, "VI Reference":refnum<vi>}[])
                n282 = call "Create_Item_List.vi"("Alias Table"=w445, "Sequence"=w453) -> ("Item List"=w454:string[])  [unwired: 1 in]
                n283 = property on="Command Sequence" class="LstBox (strict)"("Item Names"=w454) -> ()  [unwired: 2 in, 2 out]
              }
            }
          }
          event "Move Up": Value Change {
            n284 = event-data() -> ()  [unwired: 7 out]
            n285 = Current VI's Path() -> (path=w467:path)
            n286 = call "Set_Window_Saved.vi"("Saved"=FALSE, "VI Path"=w467) -> ()  [unwired: 1 out]
            n287 = property on="Command Sequence" class="LstBox (strict)"() -> ("Value"=w464:i32[])  [unwired: 2 in, 2 out]
            n288 = Sort 1D Array(array=w464) -> (sorted array=w465:i32[])
            n289 = Index Array(array=w465) -> (element=w470:i32)  [unwired: 1 in]
            n290 = Greater Than 0?(x=w470) -> (x > 0?=w471:bool)
            n291 = case shown="True" w471 {
              tunnel: w472 -> [w473 w478]
              tunnel: [w473 w475] -> w463
              tunnel: w469 -> [_ w477]
              tunnel: w465 -> [_ w476]
              frame False {
              }
              frame True {
                n292 = for {
                  tunnel: w476 -> [w480] mode=indexing
                  shift-right: [w482] -> w475
                  shift-left: w478 -> [w485]
                  tunnel: [w481] -> w474 mode=indexing
                  n293 = Decrement(x=w480) -> (x-1=w481:i32)
                  n294 = Index Array(array=w485, index #1=w480, index #2=w481) -> (element #1=w486:cluster{string, string[], dbl[], dbl}, element #2=w483:cluster{string, string[], dbl[], dbl})
                  n295 = Replace Array Subset(array=w485, new element=w486, index=w481) -> (w484:cluster{string, string[], dbl[], dbl}[])
                  n296 = Replace Array Subset(array=w484, new element=w483, index=w480) -> (w482:cluster{string, string[], dbl[], dbl}[])
                }
                n297 = call "Create_Item_List.vi"("Alias Table"=w477, "Sequence"=w475) -> ("Item List"=w479:string[])  [unwired: 1 in]
                n298 = property on="Command Sequence" class="LstBox (strict)"("Value"=w474) -> ()  [unwired: 2 in, 2 out]
                n299 = property on="Command Sequence" class="LstBox (strict)"("Item Names"=w479) -> ()  [unwired: 2 in, 2 out]
              }
            }
            n300 = call "Get_Total_Time.vi"("Input Sequence"=w463) -> ("Total Time"=w462:dbl)
            n301 = call "Seconds_To_String.vi"("Seconds"=w462) -> ("Output String"=w461:string)
            n302 = property on="Total Time" class="Str"("Value"=w461) -> ()  [unwired: 2 in, 2 out]
          }
          event "Move Down": Value Change {
            n303 = event-data() -> ()  [unwired: 7 out]
            n304 = Current VI's Path() -> (path=w494:path)
            n305 = call "Set_Window_Saved.vi"("Saved"=FALSE, "VI Path"=w494) -> ()  [unwired: 1 out]
            n306 = property on="Command Sequence" class="LstBox (strict)"() -> ("Value"=w490:i32[])  [unwired: 2 in, 2 out]
            n307 = Sort 1D Array(array=w490) -> (sorted array=w492:i32[])
            n308 = Reverse 1D Array(array=w492) -> (reversed array=w491:i32[])
            n309 = Index Array(array=w491) -> (element=w497:i32)  [unwired: 1 in]
            n310 = Array Size(array=w503) -> (size(s)=w502:i32)
            n311 = Decrement(x=w502) -> (x-1=w501:i32)
            n312 = Less?(x=w497, y=w501) -> (x < y?=w499:bool)
            n313 = Greater Or Equal To 0?(x=w497) -> (x >= 0?=w500:bool)
            n314 = And(x=w500, y=w499) -> (x .and. y?=w498:bool)
            n315 = case shown="True" w498 {
              tunnel: w503 -> [w504 w509]
              tunnel: [w504 w507] -> w489
              tunnel: w496 -> [_ w508]
              tunnel: w491 -> [_ w506]
              frame False {
              }
              frame True {
                n316 = for {
                  shift-right: [w513] -> w507
                  shift-left: w509 -> [w517]
                  tunnel: [w512] -> w505 mode=indexing
                  tunnel: w506 -> [w511] mode=indexing
                  n317 = Increment(x=w511) -> (x+1=w512:i32)
                  n318 = Index Array(array=w517, index #1=w511, index #2=w512) -> (element #1=w516:cluster{string, string[], dbl[], dbl}, element #2=w514:cluster{string, string[], dbl[], dbl})
                  n319 = Replace Array Subset(array=w517, new element=w516, index=w512) -> (w515:cluster{string, string[], dbl[], dbl}[])
                  n320 = Replace Array Subset(array=w515, new element=w514, index=w511) -> (w513:cluster{string, string[], dbl[], dbl}[])
                }
                n321 = call "Create_Item_List.vi"("Alias Table"=w508, "Sequence"=w507) -> ("Item List"=w510:string[])  [unwired: 1 in]
                n322 = property on="Command Sequence" class="LstBox (strict)"("Value"=w505) -> ()  [unwired: 2 in, 2 out]
                n323 = property on="Command Sequence" class="LstBox (strict)"("Item Names"=w510) -> ()  [unwired: 2 in, 2 out]
              }
            }
            n324 = call "Get_Total_Time.vi"("Input Sequence"=w489) -> ("Total Time"=w488:dbl)
            n325 = call "Seconds_To_String.vi"("Seconds"=w488) -> ("Output String"=w487:string)
            n326 = property on="Total Time" class="Str"("Value"=w487) -> ()  [unwired: 2 in, 2 out]
          }
          event "Preferences": Value Change {
            n327 = event-data() -> ()  [unwired: 7 out]
            n328 = call "Open_Prefs.vi"("Open Window"=TRUE) -> ("Log Files Directory Out"=w521:path, "MOCVD Database File Out"=w522:path, "Use Database Out"=w519:bool, "Cancelled"=w520:bool)
            n329 = case shown="False" w520 {
              tunnel: w522 -> [w525 _]
              tunnel: w521 -> [w527 _]
              tunnel: w519 -> [w526 _]
              frame False {
                n330 = global write "globals.vi" "Growth Database"(w525) -> ()
                "Log Files Directory" <- w527
                "Use Database" <- w526
              }
              frame True {
              }
            }
          }
          event "Set DB Info": Value Change {
            n331 = event-data() -> ()  [unwired: 7 out]
            n332 = local read "Growth Name"() -> (w529:string)
            n333 = local read "Operator Name"() -> (w530:string)
            n334 = local read "Notes"() -> (w528:string)
            n335 = call "Growth_Info_Prompt.vi"("Operator Name In"=w530, "Growth Name In"=w529, "Notes In"=w528) -> ("Operator Name Out"=w534:string, "Growth Name Out"=w533:string, "Notes Out"=w532:string, "Cancelled"=w531:bool)
            n336 = case shown="False" w531 {
              tunnel: w534 -> [w540 _]
              tunnel: w533 -> [w539 _]
              tunnel: w532 -> [w538 _]
              frame False {
                "Operator Name" <- w540
                "Growth Name" <- w539
                "Notes" <- w538
                "Db Info Set" <- TRUE ("Db Info Set")
              }
              frame True {
              }
            }
          }
          event "Command Sequence": Value Change {
            n337 = event-data() -> ("OldVal"=w548:i32[], "NewVal"=w552:i32[])  [unwired: 5 out]
            n338 = property on="opening_sequence" class="Bool (strict)"() -> ("Value"=w541:bool)  [unwired: 2 in, 2 out]
            n339 = Array Size(array=w552) -> (size(s)=w554:i32)
            n340 = case shown="False" w541 {
              tunnel: w551 -> [w567 _]
              tunnel: w550 -> [w566 w613]
              tunnel: [w565 w613] -> w549
              tunnel: w548 -> [w562 _]
              tunnel: [w558 w614] -> w546
              tunnel: w545 -> [w557 w614]
              frame False {
                n341 = property on="Delete Event" class="Bool (strict)"() -> ("Value"=w560:bool)  [unwired: 2 in, 2 out]
                n342 = Array Size(array=w562) -> (size(s)=w564:i32)
                n343 = Equal?(x=w564, y=1) -> (x = y?=w556:bool)
                n344 = Not(x=w560) -> (.not. x?=w559:bool)
                n345 = And(x=w556, y=w559) -> (x .and. y?=w561:bool)
                n346 = case shown="True" w561 {
                  tunnel: [w569 w575] -> w558
                  tunnel: w562 -> [_ w587]
                  tunnel: w557 -> [w569 w586]
                  tunnel: w567 -> [_ w582]
                  tunnel: w566 -> [w570 w581]
                  tunnel: [w570 w580] -> w565
                  tunnel: w559 -> [w568 _]
                  frame False {
                    n347 = case shown="False" w568 {
                      frame False {
                        n348 = property on="Delete Event" class="Bool (strict)"("Value"=FALSE ("Delete Event")) -> ()  [unwired: 2 in, 2 out]
                      }
                      frame True {
                      }
                    }
                  }
                  frame True {
                    n349 = Index Array(array=w587) -> (element=w574:i32)  [unwired: 1 in]
                    n350 = property on="Time (s)" class="DigNum (strict)"() -> ("NumText.Text"=w583:string)  [unwired: 2 in, 2 out]
                    n351 = Index Array(array=w586, index=w574) -> (element=w591:cluster{string, string[], dbl[], dbl})
                    n352 = Unbundle(w591) -> (w590:string)  [unwired: 3 out]
                    n353 = Fract/Exp String To Number(string=w583) -> (number=w584:dbl)  [unwired: 4 out]
                    n354 = call "Set_Time.vi"("Time"=w584, "Index"=w574, "Input Sequence"=w586) -> ("Output Sequence"=w585:cluster{string, string[], dbl[], dbl}[])
                    n355 = String Subset(string=w590, length (rest)=2 ("length (rest)")) -> (substring=w589:string)  [unwired: 1 in]
                    n356 = case shown="\"W_\"" w589 {
                      tunnel: w585 -> [w593 w598 w612]
                      tunnel: w574 -> [_ w594 w611]
                      tunnel: [w593 w596 w609] -> w579
                      tunnel: w582 -> [_ _ _]
                      tunnel: w581 -> [w592 w595 w607]
                      tunnel: [w592 w595 w607] -> w580
                      frame Default {
                      }
                      frame "R_" {
                        n357 = property on="Flow 1" class="DigNum (strict)"() -> ("NumText.Text"=w606:string)  [unwired: 2 in, 2 out]
                        n358 = property on="Flow 2" class="DigNum (strict)"() -> ("NumText.Text"=w605:string)  [unwired: 2 in, 2 out]
                        n359 = property on="Flow 3" class="DigNum (strict)"() -> ("NumText.Text"=w604:string)  [unwired: 2 in, 2 out]
                        n360 = property on="Flow 4" class="DigNum (strict)"() -> ("NumText.Text"=w603:string)  [unwired: 2 in, 2 out]
                        n361 = Fract/Exp String To Number(string=w604) -> (number=w600:dbl)  [unwired: 4 out]
                        n362 = Fract/Exp String To Number(string=w605) -> (number=w601:dbl)  [unwired: 4 out]
                        n363 = Fract/Exp String To Number(string=w603) -> (number=w599:dbl)  [unwired: 4 out]
                        n364 = Fract/Exp String To Number(string=w606) -> (number=w602:dbl)  [unwired: 4 out]
                        n365 = Build Array(w602, w601, w600, w599) -> (w597:dbl[])
                        n366 = call "Set_Flow_Array.vi"("Flow Array"=w597, "Index"=w594, "Input Sequence"=w598) -> ("Output Sequence"=w596:cluster{string, string[], dbl[], dbl}[])
                      }
                      frame "W_" {
                        n367 = call "Set_Sequence_Text_Argument.vi"("Text"="Prompt", "Argument"="Prompt", "Index"=w611, "Input Sequence"=w612) -> ("Output Sequence"=w609:cluster{string, string[], dbl[], dbl}[])  [unwired: 1 out]
                      }
                    }
                    n368 = property on="Iterations" class="DigNum (strict)"() -> ("NumText.Text"=w573:string)  [unwired: 2 in, 2 out]
                    n369 = property on="Comment" class="Str"() -> ("Value"=w578:string)  [unwired: 2 in, 2 out]
                    n370 = call "Set_Sequence_Text_Argument.vi"("Text"=w578, "Argument"="Comment", "Index"=w574, "Input Sequence"=w579) -> ("Output Sequence"=w576:cluster{string, string[], dbl[], dbl}[])  [unwired: 1 out]
                    n371 = Decimal String To Number(string=w573) -> (number=w572:i32)  [unwired: 2 in, 1 out]
                    n372 = call "Set_Iterations.vi"("Iterations"=w572, "Index"=w574, "Input Sequence"=w576) -> ("Output Sequence"=w575:cluster{string, string[], dbl[], dbl}[])
                  }
                }
              }
              frame True {
              }
            }
            n373 = Equal?(x=w554, y=1) -> (x = y?=w547:bool)
            n374 = case shown="False" w547 {
              tunnel: w546 -> [_ w659]
              tunnel: w555 -> [_ w658]
              tunnel: w552 -> [_ w650]
              tunnel: w551 -> [_ w623]
              tunnel: w546 -> [w616 w625]
              tunnel: [w616 w624] -> w542
              frame False {
                w618 = T7."Disabled and Grayed Out" ("Disabled")
                n375 = property on="Command" class="Str"("Value"="") -> ()  [unwired: 2 in, 2 out]
                n376 = property on="Command Tabs" class="TabCtl (strict)"("Value"=T1."Default" ("Command Tabs")) -> ()  [unwired: 2 in, 2 out]
                n377 = property on="Time (s)" class="DigNum (strict)"("Value"=0.0 ("Time (s)")) -> ()  [unwired: 2 in, 2 out]
                n378 = property on="Iterations" class="DigNum (strict)"("Value"=u32 1 ("Iterations")) -> ()  [unwired: 2 in, 2 out]
                n379 = property on="Comment" class="Str"("DisabledEnum"=w618) -> ()  [unwired: 2 in, 2 out]
                n380 = property on="Time (s)" class="DigNum (strict)"("DisabledEnum"=w618) -> ()  [unwired: 2 in, 2 out]
                n381 = property on="Iterations" class="DigNum (strict)"("DisabledEnum"=w618) -> ()  [unwired: 2 in, 2 out]
                n382 = property on="opening_sequence" class="Bool (strict)"("Value"=FALSE ("opening_sequence")) -> ()  [unwired: 2 in, 2 out]
              }
              frame True {
                n383 = property on="opening_sequence" class="Bool (strict)"("Value"=FALSE ("opening_sequence")) -> ()  [unwired: 2 in, 2 out]
                n384 = Index Array(array=w650) -> (element=w648:i32)  [unwired: 1 in]
                n385 = property on="Command Sequence" class="LstBox (strict)"() -> ("Value"=w657:i32[])  [unwired: 2 in, 2 out]
                n386 = Greater Or Equal To 0?(x=w648) -> (x >= 0?=w649:bool)
                n387 = case shown="True" w649 {
                  frame False {
                  }
                  frame True {
                    w666 = T7."Enabled" ("Disabled")
                    n388 = property on="Iterations" class="DigNum (strict)"("DisabledEnum"=w666) -> ()  [unwired: 2 in, 2 out]
                    n389 = property on="Comment" class="Str"("DisabledEnum"=w666) -> ()  [unwired: 2 in, 2 out]
                    n390 = property on="Time (s)" class="DigNum (strict)"("DisabledEnum"=w666) -> ()  [unwired: 2 in, 2 out]
                  }
                }
                n391 = Index Array(array=w657) -> (element=w653:i32)  [unwired: 1 in]
                n392 = call "Get_Time.vi"("Index"=w653, "Input Sequence"=w659) -> ("Time (s)"=w660:dbl)
                n393 = property on="Time (s)" class="DigNum (strict)"("Value"=w660) -> ()  [unwired: 2 in, 2 out]
                n394 = Index Array(array=w659, index=w648) -> (element=w662:cluster{string, string[], dbl[], dbl})
                n395 = Index Array(array=w659, index=w653) -> (element=w665:cluster{string, string[], dbl[], dbl})
                n396 = Unbundle(w662) -> (w630:string, w632:string[], w661:dbl[])  [unwired: 1 out]
                n397 = String Subset(string=w630, length (rest)=2 ("length (rest)")) -> (substring=w628:string)  [unwired: 1 in]
                n398 = Equal?(x="L_", y=w628) -> (x = y?=w626:bool)
                n399 = call "Get_Text_Argument.vi"("Argument"="Comment", "Argument List"=w632) -> ("Text"=w655:string)
                n400 = call "Get_Text_Argument.vi"("Argument"="API_Iterations", "Argument List"=w632) -> ("Text"=w639:string)
                n401 = property on="Comment" class="Str"("Value"=w655) -> ()  [unwired: 2 in, 2 out]
                n402 = Decimal String To Number(string=w639) -> (number=w636:i32)  [unwired: 2 in, 1 out]
                n403 = Equal To 0?(x=w636) -> (x = 0?=w638:bool)
                n404 = Unbundle(w665) -> (w656:string)  [unwired: 3 out]
                n405 = call "Get_Command_Alias.vi"("Command"=w656, "Alias Table"=w623) -> ("Alias"=→"Command":string)
                n406 = call "Get_Argument.vi"("Argument"="API_Blocking", "Argument List"=w632) -> ("Enabled"=w642:bool)
                n407 = call "Get_Argument.vi"("Argument"="API_End", "Argument List"=w632) -> ("Enabled"=w631:bool)
                n408 = And(x=w631, y=w631) -> (x .and. y?=w633:bool)
                n409 = Not(x=w631) -> (.not. x?=w634:bool)
                n410 = call "Get_Argument.vi"("Argument"="API_Wait_For_Input", "Argument List"=w632) -> ("Enabled"=w643:bool)
                n411 = Select(t=u32 1 ("Iterations"), s=w638, f=w636) -> (s? t:f=w635:u32)
                n412 = property on="Iterations" class="DigNum (strict)"("Visible"=w634) -> ()  [unwired: 2 in, 2 out]
                n413 = String Subset(string=w630, length (rest)=2 ("length (rest)")) -> (substring=w663:string)  [unwired: 1 in]
                n414 = property on="Iterations" class="DigNum (strict)"("Value"=w635) -> ()  [unwired: 2 in, 2 out]
                n415 = Or(x=w643, y=w642) -> (x .or. y?=w641:bool)
                n416 = Compound Arithmetic op=OR(w633, w641, w626) -> (w646:bool)
                n417 = Not(x=w646) -> (.not. x?=w645:bool)
                n418 = property on="Time (s)" class="DigNum (strict)"("Visible"=w645) -> ()  [unwired: 2 in, 2 out]
                n419 = case shown="\"R_\"" w663 {
                  tunnel: w632 -> [_ w672 w710 w739 w748 w758 w765]
                  tunnel: w661 -> [_ _ w732 _ _ _ _]
                  tunnel: w658 -> [_ _ w709 _ _ _ _]
                  tunnel: w630 -> [_ _ w705 _ _ _ _]
                  tunnel: w625 -> [w667 w671 w689 w736 w745 w754 w767]
                  tunnel: [w667 w670 w689 w736 w745 w754 w761] -> w624
                  tunnel: w623 -> [_ _ _ _ _ _ w762]
                  frame Default {
                    w668 = T7."Disabled and Grayed Out" ("Disabled")
                    n420 = property on="Command Tabs" class="TabCtl (strict)"("Value"=T1."Default" ("Command Tabs")) -> ()  [unwired: 2 in, 2 out]
                    n421 = property on="Comment" class="Str"("DisabledEnum"=w668) -> ()  [unwired: 2 in, 2 out]
                    n422 = property on="Time (s)" class="DigNum (strict)"("DisabledEnum"=w668) -> ()  [unwired: 2 in, 2 out]
                    n423 = property on="Iterations" class="DigNum (strict)"("DisabledEnum"=w668) -> ()  [unwired: 2 in, 2 out]
                  }
                  frame "A_" {
                    w674 = "Comment" ("Argument")
                    n424 = call "Get_Argument.vi"("Argument"="API_End", "Argument List"=w672) -> ("Enabled"=w678:bool)
                    n425 = call "Get_Text_Argument.vi"("Argument"="API_ID", "Argument List"=w672) -> ("Text"=w675:string)
                    n426 = case shown="True" w678 {
                      tunnel: [u8 0 ("Disabled") u8 2 ("Disabled")] -> w679
                      frame False {
                      }
                      frame True {
                      }
                    }
                    n427 = property on="Command Tabs" class="TabCtl (strict)"("Value"=T1."API" ("Command Tabs")) -> ()  [unwired: 2 in, 2 out]
                    n428 = call "Get_Text_Argument.vi"("Argument"=w674, "Argument List"=w672) -> ("Text"=w673:string)
                    n429 = call "Copy_Argument_For_ID.vi"("Value"=w673, "Argument"=w674, "API ID"=w675, "Input Sequence"=w671) -> ("Output Sequence"=w670:cluster{string, string[], dbl[], dbl}[])
                    n430 = property on="API Front Panel" class="Bool"("Disabled"=w679) -> ()  [unwired: 2 in, 2 out]
                  }
                  frame "R_" {
                    n431 = for {
                      tunnel: w709 -> [w735] mode=indexing
                      tunnel: [w734] -> w708 mode=indexing
                      tunnel: [w733] -> w707 mode=indexing
                      n432 = Unbundle(w735) -> (w734:string, w733:string[])
                    }
                    n433 = property on="Command Tabs" class="TabCtl (strict)"("Value"=T1."Flow" ("Command Tabs")) -> ()  [unwired: 2 in, 2 out]
                    n434 = Index Array(array=w732, index=0) -> (element=w729:dbl)
                    n435 = Search 1D Array(1D array=w708, element=w705) -> (index of element=w706:i32)  [unwired: 1 out]
                    n436 = property on="Flow 1" class="DigNum (strict)"("Value"=w729) -> ()  [unwired: 2 in, 2 out]
                    n437 = call "Get_Argument.vi"("Argument"="Active", "Argument List"=w710) -> ("Enabled"=w722:bool)
                    n438 = call "Get_Argument.vi"("Argument"="Gas_Source", "Argument List"=w710) -> ("Enabled"=w718:bool)
                    n439 = call "Get_Argument.vi"("Argument"="H2_Dilute", "Argument List"=w710) -> ("Enabled"=w684:bool)
                    n440 = Index Array(array=w707, index (row)=w706) -> (element=w690:string[])  [unwired: 1 in]
                    n441 = call "Argument_Exists.vi"("Argument"="Run", "Argument List"=w690) -> ("Argument Exists"=w703:bool)
                    n442 = property on="Active" class="Bool (strict)"("Value"=w722) -> ()  [unwired: 2 in, 2 out]
                    n443 = Index Array(array=w732, index=1) -> (element=w728:dbl)
                    n444 = property on="Gas_Source_In" class="Bool (strict)"("Value"=w718) -> ()  [unwired: 2 in, 2 out]
                    n445 = property on="H2_Dilute" class="Bool (strict)"("Value"=w684) -> ()  [unwired: 2 in, 2 out]
                    n446 = property on="Run" class="Bool (strict)"("Visible"=w703) -> ()  [unwired: 2 in, 2 out]
                    n447 = call "Argument_Exists.vi"("Argument"="Flow2", "Argument List"=w690) -> ("Argument Exists"=w687:bool)
                    n448 = call "Argument_Exists.vi"("Argument"="Flow3", "Argument List"=w690) -> ("Argument Exists"=w683:bool)
                    n449 = call "Argument_Exists.vi"("Argument"="Flow4", "Argument List"=w690) -> ()  [unwired: 1 out]
                    n450 = property on="Flow 2" class="DigNum (strict)"("Value"=w728) -> ()  [unwired: 2 in, 2 out]
                    n451 = call "Get_Argument.vi"("Argument"="H2_Flush", "Argument List"=w710) -> ("Enabled"=w713:bool)
                    n452 = property on="Flow 4" class="DigNum (strict)"("Visible"=FALSE) -> ()  [unwired: 2 in, 2 out]
                    n453 = call "Get_Argument.vi"("Argument"="Run", "Argument List"=w710) -> ("Enabled"=w720:bool)
                    n454 = And(x=w684, y=w687) -> (x .and. y?=w686:bool)
                    n455 = And(x=w684, y=w683) -> (x .and. y?=w685:bool)
                    n456 = Index Array(array=w732, index=2) -> (element=w726:dbl)
                    n457 = property on="H2 Flush" class="Bool (strict)"("Value"=w713) -> ()  [unwired: 2 in, 2 out]
                    n458 = property on="Run" class="Bool (strict)"("Value"=w720) -> ()  [unwired: 2 in, 2 out]
                    n459 = property on="Flow 2" class="DigNum (strict)"("Visible"=w686) -> ()  [unwired: 2 in, 2 out]
                    n460 = property on="Flow 3" class="DigNum (strict)"("Visible"=w685) -> ()  [unwired: 2 in, 2 out]
                    n461 = property on="Flow 3" class="DigNum (strict)"("Value"=w726) -> ()  [unwired: 2 in, 2 out]
                    n462 = Index Array(array=w732, index=3) -> (element=w724:dbl)
                    n463 = call "Argument_Exists.vi"("Argument"="H2_Flush", "Argument List"=w690) -> ("Argument Exists"=w694:bool)
                    n464 = call "Get_Argument.vi"("Argument"="Bubbler", "Argument List"=w710) -> ("Enabled"=w716:bool)
                    n465 = call "Argument_Exists.vi"("Argument"="Bubbler", "Argument List"=w690) -> ("Argument Exists"=w698:bool)
                    n466 = call "Argument_Exists.vi"("Argument"="H2_Dilute", "Argument List"=w690) -> ("Argument Exists"=w696:bool)
                    n467 = call "Argument_Exists.vi"("Argument"="Gas_Source", "Argument List"=w690) -> ("Argument Exists"=w693:bool)
                    n468 = call "Get_Argument.vi"("Argument"="Remote", "Argument List"=w710) -> ("Enabled"=w711:bool)
                    n469 = property on="H2 Flush" class="Bool (strict)"("Visible"=w694) -> ()  [unwired: 2 in, 2 out]
                    n470 = property on="Flow 4" class="DigNum (strict)"("Value"=w724) -> ()  [unwired: 2 in, 2 out]
                    n471 = property on="Bubbler In" class="Bool (strict)"("Visible"=w698) -> ()  [unwired: 2 in, 2 out]
                    n472 = property on="Gas_Source_In" class="Bool (strict)"("Visible"=w693) -> ()  [unwired: 2 in, 2 out]
                    n473 = property on="H2_Dilute" class="Bool (strict)"("Visible"=w696) -> ()  [unwired: 2 in, 2 out]
                    n474 = property on="Remote Flow" class="Bool (strict)"("Value"=w711) -> ()  [unwired: 2 in, 2 out]
                    n475 = property on="Bubbler In" class="Bool (strict)"("Value"=w716) -> ()  [unwired: 2 in, 2 out]
                  }
                  frame "H_" {
                    n476 = call "Get_Argument.vi"("Argument"="Heater", "Argument List"=w739) -> ("Enabled"=w743:bool)
                    n477 = call "Get_Argument.vi"("Argument"="Remote", "Argument List"=w739) -> ("Enabled"=w738:bool)
                    n478 = call "Get_Argument.vi"("Argument"="Spinner", "Argument List"=w739) -> ("Enabled"=w741:bool)
                    n479 = property on="Command Tabs" class="TabCtl (strict)"("Value"=T1."Heater" ("Command Tabs")) -> ()  [unwired: 2 in, 2 out]
                    n480 = property on="Heater" class="Bool (strict)"("Value"=w743) -> ()  [unwired: 2 in, 2 out]
                    n481 = property on="Spinner" class="Bool (strict)"("Value"=w741) -> ()  [unwired: 2 in, 2 out]
                    n482 = property on="Remote Heater" class="Bool (strict)"("Value"=w738) -> ()  [unwired: 2 in, 2 out]
                  }
                  frame "V_" {
                    n483 = property on="Command Tabs" class="TabCtl (strict)"("Value"=T1."Vacuum" ("Command Tabs")) -> ()  [unwired: 2 in, 2 out]
                    n484 = call "Get_Argument.vi"("Argument"="Vac_Exhaust", "Argument List"=w748) -> ("Enabled"=w752:bool)
                    n485 = call "Get_Argument.vi"("Argument"="Atm_Exhaust", "Argument List"=w748) -> ("Enabled"=w750:bool)
                    n486 = call "Get_Argument.vi"("Argument"="Remote", "Argument List"=w748) -> ("Enabled"=w747:bool)
                    n487 = property on="Remote Vacuum" class="Bool (strict)"("Value"=w747) -> ()  [unwired: 2 in, 2 out]
                    n488 = property on="Vac_Exhaust" class="Bool (strict)"("Value"=w752) -> ()  [unwired: 2 in, 2 out]
                    n489 = property on="Atm_Exhaust" class="Bool (strict)"("Value"=w750) -> ()  [unwired: 2 in, 2 out]
                  }
                  frame "W_" {
                    n490 = call "Get_Text_Argument.vi"("Argument"="Prompt", "Argument List"=w758) -> ("Text"=w756:string)
                    n491 = property on="Command Tabs" class="TabCtl (strict)"("Value"=T1."Wait" ("Command Tabs")) -> ()  [unwired: 2 in, 2 out]
                    n492 = property on="Prompt" class="Str"("Value"=w756) -> ()  [unwired: 2 in, 2 out]
                  }
                  frame "L_" {
                    w764 = "Comment" ("Argument")
                    n493 = call "Get_Text_Argument.vi"("Argument"="API_ID", "Argument List"=w765) -> ("Text"=w766:string)
                    n494 = call "Get_Text_Argument.vi"("Argument"=w764, "Argument List"=w765) -> ("Text"=w763:string)
                    n495 = property on="Command Tabs" class="TabCtl (strict)"("Value"=T1."Default" ("Command Tabs")) -> ()  [unwired: 2 in, 2 out]
                    n496 = call "Copy_Argument_For_ID.vi"("Value"=w763, "Argument"=w764, "API ID"=w766, "Input Sequence"=w767) -> ("Output Sequence"=w761:cluster{string, string[], dbl[], dbl}[])
                    n497 = call "Create_Item_List.vi"("Alias Table"=w762, "Sequence"=w761) -> ("Item List"=w760:string[])  [unwired: 1 in]
                    n498 = property on="Command Sequence" class="LstBox (strict)"("Item Names"=w760) -> ()  [unwired: 2 in, 2 out]
                  }
                }
              }
            }
            n499 = call "Get_Total_Time.vi"("Input Sequence"=w542) -> ("Total Time"=w543:dbl)
            n500 = call "Seconds_To_String.vi"("Seconds"=w543) -> ("Output String"=→"Total Time":string)
          }
          event "Time (s)": Value Change {
            n501 = event-data() -> ()  [unwired: 7 out]
            n502 = property on="Command Sequence" class="LstBox (strict)"() -> ("Value"=w773:i32[])  [unwired: 2 in, 2 out]
            n503 = property on="Command Sequence" class="LstBox (strict)"("Val(Sgnl)"=w773) -> ()  [unwired: 2 in, 2 out]
            n504 = Current VI's Path() -> (path=w770:path)
            n505 = call "Set_Window_Saved.vi"("Saved"=FALSE, "VI Path"=w770) -> ()  [unwired: 1 out]
          }
          event "Iterations": Value Change {
            n506 = event-data() -> ()  [unwired: 7 out]
            n507 = property on="Command Sequence" class="LstBox (strict)"() -> ("Value"=w775:i32[])  [unwired: 2 in, 2 out]
            n508 = property on="Command Sequence" class="LstBox (strict)"("Val(Sgnl)"=w775) -> ()  [unwired: 2 in, 2 out]
            n509 = Current VI's Path() -> (path=w777:path)
            n510 = call "Set_Window_Saved.vi"("Saved"=FALSE, "VI Path"=w777) -> ()  [unwired: 1 out]
          }
          event "Comment": Value Change {
            n511 = event-data() -> ()  [unwired: 7 out]
            n512 = property on="Command Sequence" class="LstBox (strict)"() -> ("Value"=w779:i32[])  [unwired: 2 in, 2 out]
            n513 = property on="Command Sequence" class="LstBox (strict)"("Val(Sgnl)"=w779) -> ()  [unwired: 2 in, 2 out]
            n514 = Current VI's Path() -> (path=w781:path)
            n515 = call "Set_Window_Saved.vi"("Saved"=FALSE, "VI Path"=w781) -> ()  [unwired: 1 out]
          }
          event "Flow 1", "Flow 2", "Flow 3", "Flow 4": Value Change {
            n516 = event-data() -> ()  [unwired: 7 out]
            n517 = property on="Command Sequence" class="LstBox (strict)"() -> ("Value"=w788:i32[])  [unwired: 2 in, 2 out]
            n518 = property on="Command Sequence" class="LstBox (strict)"("Val(Sgnl)"=w788) -> ()  [unwired: 2 in, 2 out]
            n519 = Current VI's Path() -> (path=w785:path)
            n520 = call "Set_Window_Saved.vi"("Saved"=FALSE, "VI Path"=w785) -> ()  [unwired: 1 out]
          }
          event "Remote Flow": Value Change {
            n521 = event-data() -> ()  [unwired: 7 out]
            n522 = Current VI's Path() -> (path=w790:path)
            n523 = call "Set_Window_Saved.vi"("Saved"=FALSE, "VI Path"=w790) -> ()  [unwired: 1 out]
            n524 = property on="Command Sequence" class="LstBox (strict)"() -> ("Value"=w793:i32[])  [unwired: 2 in, 2 out]
            n525 = Index Array(array=w793) -> (element=w792:i32)  [unwired: 1 in]
            n526 = call "Set_Sequence_Argument.vi"("Enable"="Remote Flow", "Argument"="Remote", "Index"=w792, "Input Sequence"=w797) -> ("Output Sequence"=w795:cluster{string, string[], dbl[], dbl}[])  [unwired: 1 out]
          }
          event "Remote Heater": Value Change {
            n527 = event-data() -> ()  [unwired: 7 out]
            n528 = Current VI's Path() -> (path=w799:path)
            n529 = call "Set_Window_Saved.vi"("Saved"=FALSE, "VI Path"=w799) -> ()  [unwired: 1 out]
            n530 = property on="Command Sequence" class="LstBox (strict)"() -> ("Value"=w802:i32[])  [unwired: 2 in, 2 out]
            n531 = Index Array(array=w802) -> (element=w801:i32)  [unwired: 1 in]
            n532 = call "Set_Sequence_Argument.vi"("Enable"="Remote Heater", "Argument"="Remote", "Index"=w801, "Input Sequence"=w806) -> ("Output Sequence"=w804:cluster{string, string[], dbl[], dbl}[])  [unwired: 1 out]
          }
          event "Remote Vacuum": Value Change {
            n533 = event-data() -> ()  [unwired: 7 out]
            n534 = Current VI's Path() -> (path=w808:path)
            n535 = call "Set_Window_Saved.vi"("Saved"=FALSE, "VI Path"=w808) -> ()  [unwired: 1 out]
            n536 = property on="Command Sequence" class="LstBox (strict)"() -> ("Value"=w811:i32[])  [unwired: 2 in, 2 out]
            n537 = Index Array(array=w811) -> (element=w810:i32)  [unwired: 1 in]
            n538 = call "Set_Sequence_Argument.vi"("Enable"="Remote Vacuum", "Argument"="Remote", "Index"=w810, "Input Sequence"=w815) -> ("Output Sequence"=w813:cluster{string, string[], dbl[], dbl}[])  [unwired: 1 out]
          }
          event "Active": Value Change {
            n539 = event-data() -> ()  [unwired: 7 out]
            n540 = Current VI's Path() -> (path=w817:path)
            n541 = call "Set_Window_Saved.vi"("Saved"=FALSE, "VI Path"=w817) -> ()  [unwired: 1 out]
            n542 = property on="Command Sequence" class="LstBox (strict)"() -> ("Value"=w820:i32[])  [unwired: 2 in, 2 out]
            n543 = Index Array(array=w820) -> (element=w819:i32)  [unwired: 1 in]
            n544 = call "Set_Sequence_Argument.vi"("Enable"="Active", "Argument"="Active", "Index"=w819, "Input Sequence"=w824) -> ("Output Sequence"=w822:cluster{string, string[], dbl[], dbl}[])  [unwired: 1 out]
          }
          event "Run": Value Change {
            n545 = event-data() -> ()  [unwired: 7 out]
            n546 = Current VI's Path() -> (path=w826:path)
            n547 = call "Set_Window_Saved.vi"("Saved"=FALSE, "VI Path"=w826) -> ()  [unwired: 1 out]
            n548 = property on="Command Sequence" class="LstBox (strict)"() -> ("Value"=w829:i32[])  [unwired: 2 in, 2 out]
            n549 = Index Array(array=w829) -> (element=w828:i32)  [unwired: 1 in]
            n550 = call "Set_Sequence_Argument.vi"("Enable"="Run", "Argument"="Run", "Index"=w828, "Input Sequence"=w833) -> ("Output Sequence"=w831:cluster{string, string[], dbl[], dbl}[])  [unwired: 1 out]
          }
          event "Gas_Source_In": Value Change {
            n551 = event-data() -> ()  [unwired: 7 out]
            n552 = Current VI's Path() -> (path=w835:path)
            n553 = call "Set_Window_Saved.vi"("Saved"=FALSE, "VI Path"=w835) -> ()  [unwired: 1 out]
            n554 = property on="Command Sequence" class="LstBox (strict)"() -> ("Value"=w838:i32[])  [unwired: 2 in, 2 out]
            n555 = Index Array(array=w838) -> (element=w837:i32)  [unwired: 1 in]
            n556 = call "Set_Sequence_Argument.vi"("Enable"="Gas_Source_In", "Argument"="Gas_Source", "Index"=w837, "Input Sequence"=w842) -> ("Output Sequence"=w840:cluster{string, string[], dbl[], dbl}[])  [unwired: 1 out]
          }
          event "H2 Flush": Value Change {
            n557 = event-data() -> ()  [unwired: 7 out]
            n558 = Current VI's Path() -> (path=w844:path)
            n559 = call "Set_Window_Saved.vi"("Saved"=FALSE, "VI Path"=w844) -> ()  [unwired: 1 out]
            n560 = property on="Command Sequence" class="LstBox (strict)"() -> ("Value"=w847:i32[])  [unwired: 2 in, 2 out]
            n561 = Index Array(array=w847) -> (element=w846:i32)  [unwired: 1 in]
            n562 = call "Set_Sequence_Argument.vi"("Enable"="H2 Flush", "Argument"="H2_Flush", "Index"=w846, "Input Sequence"=w851) -> ("Output Sequence"=w849:cluster{string, string[], dbl[], dbl}[])  [unwired: 1 out]
          }
          event "Bubbler In": Value Change {
            n563 = event-data() -> ()  [unwired: 7 out]
            n564 = Current VI's Path() -> (path=w853:path)
            n565 = call "Set_Window_Saved.vi"("Saved"=FALSE, "VI Path"=w853) -> ()  [unwired: 1 out]
            n566 = property on="Command Sequence" class="LstBox (strict)"() -> ("Value"=w856:i32[])  [unwired: 2 in, 2 out]
            n567 = Index Array(array=w856) -> (element=w855:i32)  [unwired: 1 in]
            n568 = call "Set_Sequence_Argument.vi"("Enable"="Bubbler In", "Argument"="Bubbler", "Index"=w855, "Input Sequence"=w860) -> ("Output Sequence"=w858:cluster{string, string[], dbl[], dbl}[])  [unwired: 1 out]
          }
          event "H2_Dilute": Value Change {
            n569 = event-data() -> ()  [unwired: 7 out]
            n570 = Current VI's Path() -> (path=w863:path)
            n571 = call "Set_Window_Saved.vi"("Saved"=FALSE, "VI Path"=w863) -> ()  [unwired: 1 out]
            n572 = property on="Command Sequence" class="LstBox (strict)"() -> ("Value"=w861:i32[])  [unwired: 2 in, 2 out]
            n573 = property on="Command Sequence" class="LstBox (strict)"() -> ("Value"=w866:i32[])  [unwired: 2 in, 2 out]
            n574 = property on="Command Sequence" class="LstBox (strict)"("Val(Sgnl)"=w861) -> ()  [unwired: 2 in, 2 out]
            n575 = Index Array(array=w866) -> (element=w865:i32)  [unwired: 1 in]
            n576 = call "Set_Sequence_Argument.vi"("Enable"="H2_Dilute", "Argument"="H2_Dilute", "Index"=w865, "Input Sequence"=w870) -> ("Output Sequence"=w868:cluster{string, string[], dbl[], dbl}[])  [unwired: 1 out]
          }
          event "Heater": Value Change {
            n577 = event-data() -> ()  [unwired: 7 out]
            n578 = Current VI's Path() -> (path=w872:path)
            n579 = call "Set_Window_Saved.vi"("Saved"=FALSE, "VI Path"=w872) -> ()  [unwired: 1 out]
            n580 = property on="Command Sequence" class="LstBox (strict)"() -> ("Value"=w875:i32[])  [unwired: 2 in, 2 out]
            n581 = Index Array(array=w875) -> (element=w874:i32)  [unwired: 1 in]
            n582 = call "Set_Sequence_Argument.vi"("Enable"="Heater", "Argument"="Heater", "Index"=w874, "Input Sequence"=w879) -> ("Output Sequence"=w877:cluster{string, string[], dbl[], dbl}[])  [unwired: 1 out]
          }
          event "Spinner": Value Change {
            n583 = event-data() -> ()  [unwired: 7 out]
            n584 = Current VI's Path() -> (path=w881:path)
            n585 = call "Set_Window_Saved.vi"("Saved"=FALSE, "VI Path"=w881) -> ()  [unwired: 1 out]
            n586 = property on="Command Sequence" class="LstBox (strict)"() -> ("Value"=w884:i32[])  [unwired: 2 in, 2 out]
            n587 = Index Array(array=w884) -> (element=w883:i32)  [unwired: 1 in]
            n588 = call "Set_Sequence_Argument.vi"("Enable"="Spinner", "Argument"="Spinner", "Index"=w883, "Input Sequence"=w888) -> ("Output Sequence"=w886:cluster{string, string[], dbl[], dbl}[])  [unwired: 1 out]
          }
          event "Vac_Exhaust": Value Change {
            n589 = event-data() -> ()  [unwired: 7 out]
            n590 = Current VI's Path() -> (path=w890:path)
            n591 = call "Set_Window_Saved.vi"("Saved"=FALSE, "VI Path"=w890) -> ()  [unwired: 1 out]
            n592 = property on="Command Sequence" class="LstBox (strict)"() -> ("Value"=w893:i32[])  [unwired: 2 in, 2 out]
            n593 = Index Array(array=w893) -> (element=w892:i32)  [unwired: 1 in]
            n594 = call "Set_Sequence_Argument.vi"("Enable"="Vac_Exhaust", "Argument"="Vac_Exhaust", "Index"=w892, "Input Sequence"=w897) -> ("Output Sequence"=w895:cluster{string, string[], dbl[], dbl}[])  [unwired: 1 out]
          }
          event "Atm_Exhaust": Value Change {
            n595 = event-data() -> ()  [unwired: 7 out]
            n596 = Current VI's Path() -> (path=w899:path)
            n597 = call "Set_Window_Saved.vi"("Saved"=FALSE, "VI Path"=w899) -> ()  [unwired: 1 out]
            n598 = property on="Command Sequence" class="LstBox (strict)"() -> ("Value"=w902:i32[])  [unwired: 2 in, 2 out]
            n599 = Index Array(array=w902) -> (element=w901:i32)  [unwired: 1 in]
            n600 = call "Set_Sequence_Argument.vi"("Enable"="Atm_Exhaust", "Argument"="Atm_Exhaust", "Index"=w901, "Input Sequence"=w906) -> ("Output Sequence"=w904:cluster{string, string[], dbl[], dbl}[])  [unwired: 1 out]
          }
          event "Prompt": Value Change {
            n601 = event-data() -> ()  [unwired: 7 out]
            n602 = property on="Command Sequence" class="LstBox (strict)"() -> ("Value"=w910:i32[])  [unwired: 2 in, 2 out]
            n603 = property on="Command Sequence" class="LstBox (strict)"("Val(Sgnl)"=w910) -> ()  [unwired: 2 in, 2 out]
            n604 = Current VI's Path() -> (path=w908:path)
            n605 = call "Set_Window_Saved.vi"("Saved"=FALSE, "VI Path"=w908) -> ()  [unwired: 1 out]
          }
          event "API Front Panel": Value Change {
            n606 = event-data() -> ()  [unwired: 7 out]
            n607 = property on="Command Sequence" class="LstBox (strict)"() -> ("Value"=w933:i32[])  [unwired: 2 in, 2 out]
            n608 = Index Array(array=w933) -> (element=w932:i32)  [unwired: 1 in]
            n609 = Index Array(array=w935, index=w932) -> (element=w938:cluster{string, string[], dbl[], dbl})
            n610 = Unbundle(w938) -> (w937:string, w912:string[], w936:dbl[], w922:dbl)
            n611 = call "Get_API_Mode.vi"("Argument List"=w912) -> ("API Mode"=w913:T5)
            n612 = case shown="\"Finite\"" w913 {
              tunnel: [w939 w942] -> w914
              tunnel: w912 -> [w939 w943]
              frame Default {
              }
              frame "Finite" {
                n613 = property on="Time (s)" class="DigNum (strict)"() -> ("Value"=w941:dbl)  [unwired: 2 in, 2 out]
                n614 = call "SetNumberArgument.vi"("value"=w941, "Argument"="API_Calculated_Time", "Argument List In"=w943) -> ("Argument List Out"=w942:string[])  [unwired: 1 out]
              }
            }
            n615 = call "API_Call.vi"("API Function Array"=w931, "Argument List In"=w914, "State"=enum16{"Edit", "Start", "Run", "End", "Idle"}."Edit") -> ("Argument List Out"=w916:string[])  [unwired: 2 in, 1 out]
            n616 = Array Size(array=w916) -> (size(s)=w918:i32)
            n617 = Equal To 0?(x=w918) -> (x = 0?=w917:bool)
            n618 = case shown="True" w917 {
              tunnel: w916 -> [w944 _]
              tunnel: w912 -> [_ w945]
              tunnel: [w944 w945] -> w915
              frame False {
              }
              frame True {
              }
            }
            n619 = Not Equal?(x=w912, y=w915) -> (x != y?=w925:bool)
            n620 = case shown="True" w925 {
              frame False {
              }
              frame True {
                n621 = Current VI's Path() -> (path=w950:path)
                n622 = call "Set_Window_Saved.vi"("Saved"=FALSE, "VI Path"=w950) -> ()  [unwired: 1 out]
              }
            }
            n623 = call "Get_Text_Argument.vi"("Argument"="API_Calculated_Time", "Argument List"=w915) -> ("Text"=w921:string)
            n624 = Not Equal?(x=w921, y="") -> (x != y?=w919:bool)
            n625 = case shown="False" w919 {
              tunnel: [w946 w947] -> w923
              tunnel: w922 -> [w946 _]
              tunnel: w921 -> [_ w948]
              frame False {
              }
              frame True {
                n626 = Fract/Exp String To Number(string=w948) -> (number=w947:dbl)  [unwired: 3 in, 1 out]
                n627 = property on="Time (s)" class="DigNum (strict)"("Val(Sgnl)"=w947) -> ()  [unwired: 2 in, 2 out]
              }
            }
            n628 = Bundle(w937, "Argument List Out"=w915, w936, w923) -> (w926:T6)  [unwired: 1 out]
            n629 = Replace Array Subset(array=w935, new element=w926, index=w932) -> (w928:cluster{string, string[], dbl[], dbl}[])
            n630 = call "Copy_API_Description.vi"("Event"=w926, "Input Sequence"=w928) -> ("Output Sequence"=w927:cluster{string, string[], dbl[], dbl}[])
            n631 = call "Create_Item_List.vi"("Alias Table"=w930, "Sequence"=w927) -> ("Item List"=w929:string[])  [unwired: 1 in]
            n632 = property on="Command Sequence" class="LstBox (strict)"("Item Names"=w929) -> ()  [unwired: 2 in, 2 out]
          }
          event "View Log": Value Change {
            n633 = event-data() -> ()  [unwired: 7 out]
            n634 = call "View_Log.vi"() -> ()  [unwired: 12 out]
          }
          event "Run Sequence": Value Change {
            n635 = event-data() -> ()  [unwired: 7 out]
            n636 = local read "Use Database"() -> (w960:bool)
            n637 = local read "Db Info Set"() -> (w959:bool)
            n638 = property on="Operating Mode" class="RadioBtnsControl (strict)"() -> ("Value"=w962:enum32{"Production", "Debug"})  [unwired: 2 in, 2 out]
            n639 = Equal?(x=w962, y=enum32{"Production", "Debug"}."Production") -> (x = y?=w953:bool)
            n640 = Compound Arithmetic op=AND(w953, w960, w959) -> (w958:bool)
            n641 = case shown="True" w958 {
              tunnel: [w974 w975] -> w954
              tunnel: w955 -> [w974 w975]
              frame False {
                n642 = global write "globals.vi" "Log Path"(path "") -> ()
              }
              frame True {
                n643 = local read "Current File Path"() -> (w977:path)
                n644 = local read "Operator Name"() -> (w982:string)
                n645 = local read "Growth Name"() -> (w981:string)
                n646 = local read "Notes"() -> (w980:string)
                n647 = Not Equal?(x=w977, y=path "") -> (x != y?=w978:bool)
                n648 = case shown="True" w978 {
                  tunnel: [w987 w990] -> w986
                  tunnel: w977 -> [_ w991]
                  frame False {
                    n649 = call "Get_Timestamp.vi"() -> ("Timestamp"=w989:string)  [unwired: 1 in]
                    n650 = Concatenate Strings(w989, ".log" ("string")) -> (w987:string)
                  }
                  frame True {
                    n651 = Strip Path(path=w991) -> (name=w990:string)  [unwired: 1 out]
                  }
                }
                n652 = local read "Log Files Directory"() -> (w983:path)
                n653 = Build Path(base path=w983, name or relative path=w986) -> (appended path=w984:path)
                n654 = call "Write_Growth_DB.vi"("Growth Name"=w981, "Notes"=w980, "Log File"=w977, "Growth Sequence File"=w984, "Operator Name"=w982) -> ("Error"=w976:bool)
                n655 = case shown="True" w976 {
                  tunnel: "Warning: Could not write to growth database" ("message") -> [_ w992]
                  frame False {
                  }
                  frame True {
                    n656 = One Button Dialog(message=w992) -> ()  [unwired: 1 in, 1 out]
                  }
                }
                n657 = global write "globals.vi" "Log Path"(w984) -> ()
              }
            }
            n658 = call "Check_Sequence.vi"("Input Sequence"=w954) -> ("Valid Sequence"=w957:bool, "Error Indices"=w956:i32[])
            n659 = case shown="True" w957 {
              tunnel: w964 -> [_ w970]
              tunnel: w956 -> [w965 _]
              frame False {
                n660 = property on="Command Sequence" class="LstBox (strict)"("Val(Sgnl)"=w965) -> ()  [unwired: 2 in, 2 out]
              }
              frame True {
                n661 = Two Button Dialog(message="Confirm and begin sequence?", 1:"Cancel" ("F button name (\"Cancel\")"), 2:"OK" ("T button name (\"OK\")")) -> (T button?=w966:bool)
                n662 = case shown="True" w966 {
                  tunnel: w970 -> [_ w972]
                  frame False {
                  }
                  frame True {
                    n663 = Generate User Event(user event=w972, event data cluster=cluster{"Resume":bool, "Start Event":i32} {"Resume"=FALSE, "Start Event"=0} ("event data")) -> ()  [unwired: 1 in, 2 out]
                  }
                }
              }
            }
          }
          event "Resume": Value Change {
            n664 = event-data() -> ()  [unwired: 7 out]
            n665 = call "Check_Sequence.vi"("Input Sequence"=w995) -> ("Valid Sequence"=w994:bool, "Error Indices"=w993:i32[])
            n666 = property on="Command Sequence" class="LstBox (strict)"("Val(Sgnl)"=w993) -> ()  [unwired: 2 in, 2 out]
            n667 = case shown="True" w994 {
              tunnel: [FALSE w1005] -> w1000
              tunnel: [_ w1004] -> w998
              tunnel: w997 -> [_ w1003]
              tunnel: w995 -> [_ w1002]
              frame False {
              }
              frame True {
                n668 = call "Resume_Sequence.vi"("Alias Table"=w1003, "Sequence"=w1002) -> ("Cancelled"=w1006:bool, "Start Event Value"=w1004:i32)
                n669 = Not(x=w1006) -> (.not. x?=w1005:bool)
              }
            }
            n670 = case shown="True" w1000 {
              tunnel: w999 -> [_ w1010]
              tunnel: w998 -> [_ w1007]
              frame False {
              }
              frame True {
                n671 = Bundle(TRUE, "Start Event Value"=w1007) -> (w1009:cluster{bool, "Start Event Value":i32})  [unwired: 1 out]
                n672 = Generate User Event(user event=w1010, event data cluster=w1009) -> ()  [unwired: 1 in, 2 out]
              }
            }
          }
          event User Event {
            n673 = event-data() -> ("Resume"=w1012:bool, "Start Event"=w1017:i32)  [unwired: 5 out]
            n674 = case shown="True" w1012 {
              tunnel: w1018 -> [w1021 w1025]
              tunnel: w1017 -> [_ w1023]
              tunnel: [w1021 w1022] -> w1016
              frame False {
              }
              frame True {
                n675 = Delete From Array(array=w1025, length=w1023, index=0) -> (array with subset deleted=w1022:cluster{string, string[], dbl[], dbl}[])  [unwired: 1 out]
              }
            }
            n676 = case shown="\"Production\"" "Operating Mode" {
              tunnel: [FALSE TRUE] -> w1014
              frame "Production" {
              }
              frame "Debug", Default {
              }
            }
            n677 = call "Run_Sequence.vi"("Input Sequence"=w1016, "Alias Table"=w1013, "API Function Array"=w1011, "Debug"=w1014, "Resume"=w1012) -> ()  [unwired: 1 out]
          }
        }
      }
    }
  }
